vi "sub_peltier 1 control.vi"(0 "Save File":path, 1 "Save Data to File":bool caption="Save?", 3 "COM":i16, 4 "Array #":i32) -> ()   [LabVIEW 2020]
uses:
  <vilib>/Instr/_visa.llb/VISA Find Search Mode.ctl
  <vilib>/Utility/error.llb/DialogType.ctl
  globalvariables.vi
  <vilib>/Utility/file.llb/Write Delimited Spreadsheet (string).vi
  <vilib>/Utility/file.llb/Write Delimited Spreadsheet (DBL).vi
panel:
  in  "Controller Settings":enum32{"Page 1"}(tab)
  in  "Proportional Bandwidth":dbl=50.0
  in  "Integral Gain":dbl
  in  "Derivative Gain":dbl
  in  "Set Limit High":dbl=100.0
  in  "Set Limit Low":dbl=-20.0
  in  "Control Sensor Offset":dbl
  in  "Sample Rate (s)":i16=1
  in  "Alarm Settings":enum32{"Page 1"}(tab)
  in  "Shutdown Output w/ Alarm 2":bool
  in  "Clear Alarm Latch":bool
  in  "Shutdown Output w/ Alarm 1":bool
  in  "Alarm 2 Deadband":dbl
  in  "Alarm 2 Low":dbl
  in  "Alarm 2 High":dbl=60.0
  in  "Alarm 1 Deadband":dbl
  in  "Alarm 1 Low":dbl
  in  "Alarm 1 High":dbl=60.0
  in  "Alarm Latch":T1(radio)
  out "Alarm":bool
  in  "Graph Data":enum32{"Tab 1"}(tab)
  in  "About":bool
  out "Elapsed Time":dbl=-3262346310.140625
  out "Start Sample Time":timestamp=timestamp(3262346310.140625 s since 1904-01-01)
  out "Sample in Time":timestamp
  in  "Strip Chart 2":T2={"TEMPERATURE"=36.2, "Value"=-16.0, "Value 2"=-13.8}
  out "Set Temperature":dbl
  out "Input 2 Sensor":dbl
  out "Control Sensor":dbl
  in  "Misc Settings":enum32{"Page 1"}(tab)
  in  "Analog Output Multiplier":dbl=1.0
  in  "Sensor Type":enum32{"15K", "10K"}(radio)=enum."10K"
  in  "Output Polarity":enum32{"Cool", "Heat "}(radio)
  in  "EEPROM Write Enable":bool
  in  "Temperature 2 Display":T3(radio)=enum."Radio Selection 3"
  out "Firmware Version":string
  out "CRC Error":bool
  out "error out":errorcluster
  out "Reading Configuration":sgl
  in  "Tab Control":enum32{"Page 1"}(tab)
  out "Power":i16(slide) scale=0.0..100.0
  out "Strip Chart":T2(graph)
  out "Sampling":bool
  in  "Run Peltier":bool
  # "%"
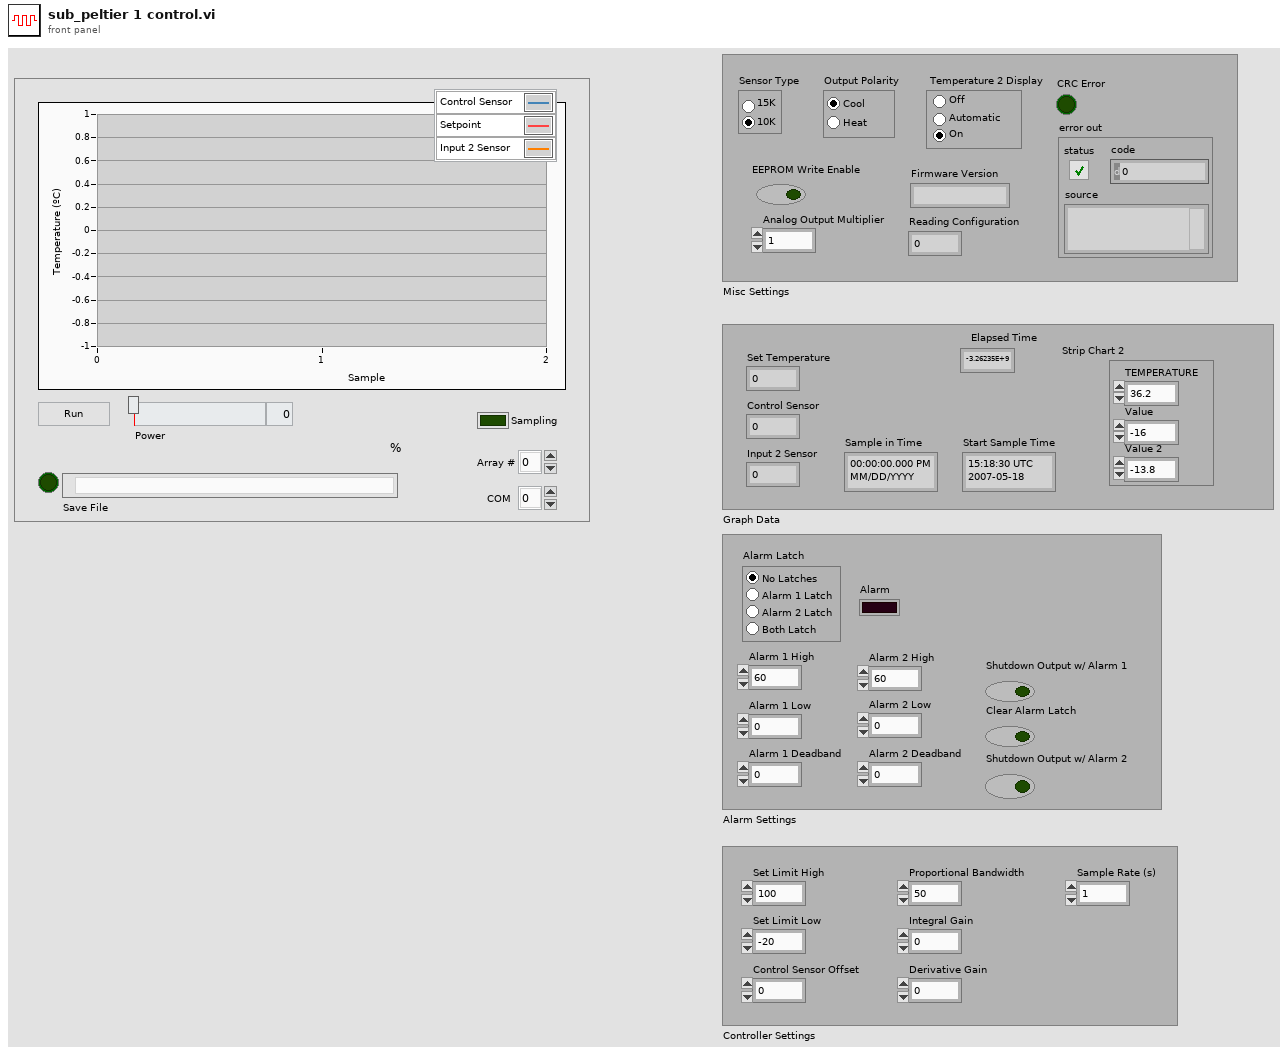
[diagram p1: front panel]
types:
  T1 = enum32{"Radio Selection 1", "Radio Selection 2", "Radio Selection 3", "Radio Selection 4"}
  T2 = cluster{"TEMPERATURE":dbl, "Value":dbl, "Value 2":dbl}
  T3 = enum32{"Radio Selection 1", "Radio Selection 2", "Radio Selection 3"}
  T4 = cluster{"Read Model":bool, "Read Settings":bool, "Read Controls":bool, "Sample":bool, "Start":bool, "End":bool, "CRC Error":bool}
  T5 = typedef "VISA Find Search Mode.ctl" = u32
  T6 = cluster{"TEMPERATURE":dbl, "Value":dbl, "Value 2":dbl}[]
  T7 = typedef "DialogType.ctl" = u16
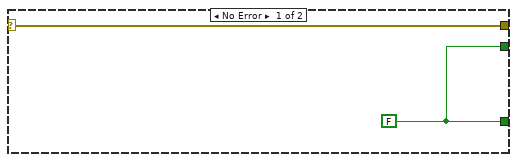
[diagram p2: hidden frame]
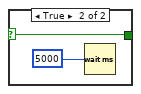
[diagram p3: hidden frame]
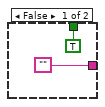
[diagram p4: hidden frame]
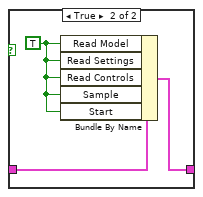
[diagram p10: hidden frame]
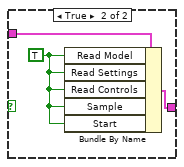
[diagram p12: hidden frame]
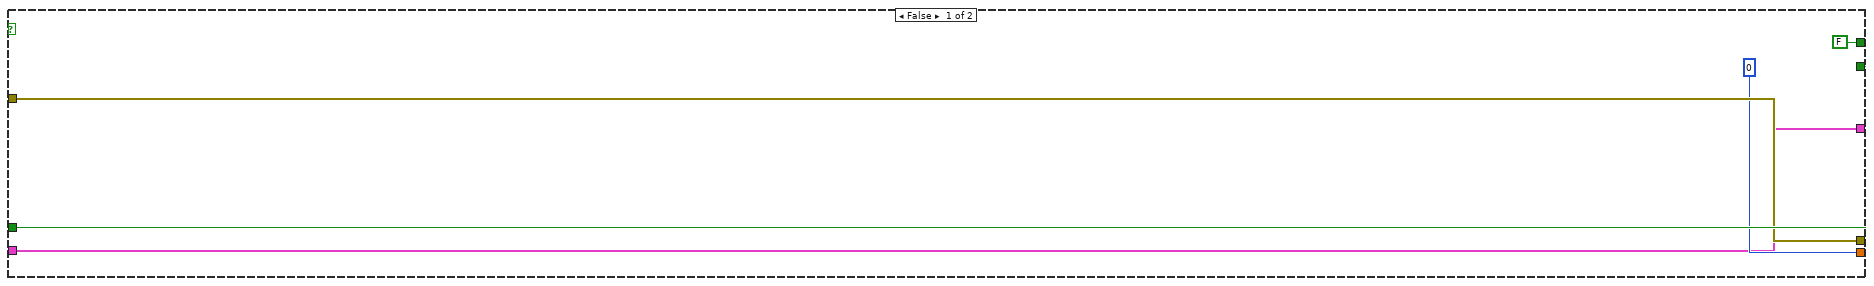
[diagram p13: hidden frame]
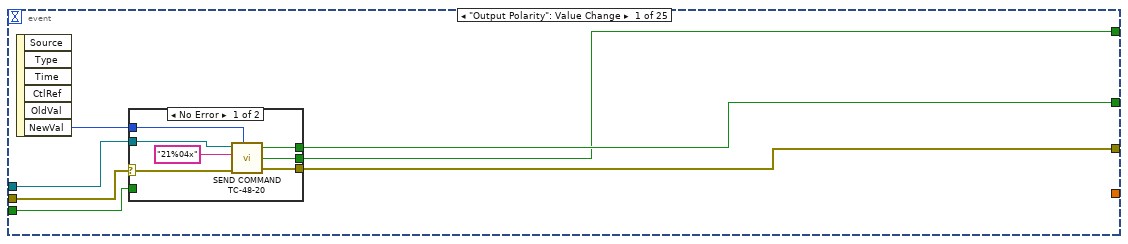
[diagram p16: hidden frame]
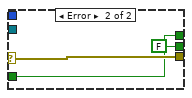
[diagram p17: hidden frame]
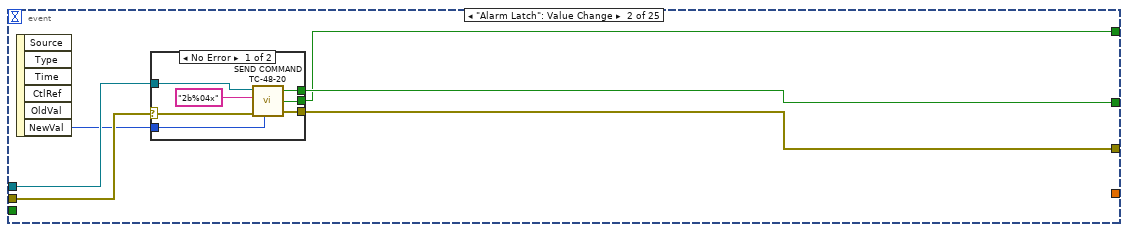
[diagram p18: hidden frame]
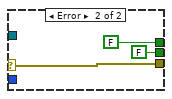
[diagram p19: hidden frame]
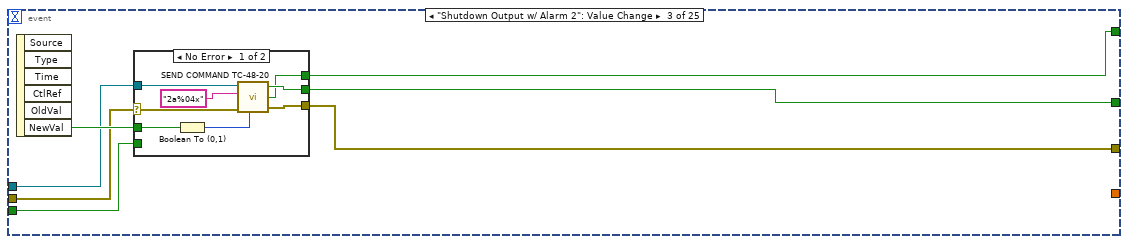
[diagram p20: hidden frame]
diagram:
  w1 = FALSE  # CRC Error
  w2 = FALSE  # End
  w4 = TRUE  # Start
  w5 = TRUE  # Sample
  w6 = TRUE  # Read Controls
  w7 = TRUE  # Read Settings
  w8 = TRUE  # Read Model
  # "CHECK CONTROLS"
  n1 = Bundle("Read Model"=w8, "Read Settings"=w7, "Read Controls"=w6, "Sample"=w5, "Start"=w4, "End"=w2, "CRC Error"=w1) -> (w3:T4)  [unwired: 1 in]
  n2 = while {
    tunnel: [w24] -> w12
    tunnel: [w19] -> w11
    tunnel: errorcluster {"status"=FALSE, "code"=0, "source"=""} ("Startup error in (no error)") -> [w23]
    tunnel: w3 -> [w17]
    tunnel: [w14] -> w10
    stop <- w18 continue-if-true
    # "Connect to Peltier Controller"
    n3 = while {
      tunnel: w23 -> [w46]
      tunnel: [w48] -> w22
      tunnel: [w50] -> w21
      tunnel: [w39] -> w16
      stop <- TRUE stop-if-true
      w55 = u16 0 items=["None", "XON/XOFF", "RTS/CTS", "XON/XOFF & RTS/CTS", "DTR/DSR", "XON/XOFF & DTR/DSR"] ("Serial Settings:Flow Control")
      w51 = u16 0 items=["None", "Odd", "Even", "Mark", "Space"] ("Serial Settings:Parity")
      w56 = T5 4 items=["Canonical Names Only"=0, "Aliases Only"=1, "Include Matching Aliases"=2, "Include All Aliases"=4] ("Search Mode")
      n4 = Greater Than 0?(x="COM") -> (x > 0?=w42:bool)
      n5 = property on="Firmware Version" class="Str"("Value"="") -> ()  [unwired: 2 in, 2 out]
      n6 = case shown="True" w42 {
        tunnel: "COM" -> [_ w63]
        tunnel: ["" w60] -> w40
        tunnel: [TRUE FALSE] -> w39
        frame False {
        }
        frame True {
          n7 = Number To Decimal String(number=w63) -> (decimal integer string=w61:string)  [unwired: 1 in]
          n8 = Concatenate Strings("COM", w61) -> (w60:string)
        }
      }
      n9 = VISA Find Resource(8:w46, 10:w56) -> (0:w49:errorcluster)  [unwired: 1 in, 2 out]
      n10 = Coerce To Type(0:w40, 1:refnum<visa-resource-name> refnum ("SELECT PORT")) -> (2:w43:refnum<visa-resource-name>)
      n11 = property class="Instr" props=["Baud", "Data Bits", "Parity", "Stop Bits", "Flow Cntrl", "Rsrc Name", "Is Connected"](reference=w43, error in=w49, "Baud"=u32 115200 ("Numeric 6"), "Data Bits"=u16 8, "Parity"=w51, "Stop Bits"=u16 10, "Flow Cntrl"=w55) -> (reference out=w50:refnum<visa-resource-name>, error out=w48:errorcluster)  [unwired: 2 out]
    }
    n12 = VISA Set I/O Buffer Size(VISA resource name=w21, error in (no error)=w22) -> (VISA resource name out=w25:refnum<visa-resource-name>, error out=w26:errorcluster)  [unwired: 2 in]
    n13 = VISA Flush I/O Buffer(VISA resource name=w25, error in (no error)=w26) -> (VISA resource name out=w24:refnum<visa-resource-name>, error out=w20:errorcluster)  [unwired: 1 in]
    n14 = case shown="Error" w20 {
      selector: w20 -> [w28 w32]
      tunnel: [w28 w32] -> w19
      tunnel: [w27 w30] -> w18
      tunnel: [w27 w29] -> w15
      frame No Error {
        w27 = FALSE
      }
      frame Error {
        n15 = Two Button Dialog(message=" Unable to communicate with controller (Error 1), check:\n• Controller is ON and correctly wired\n• Correct communications port is selected\n• Another program is not using the communications port ", 1:"EXIT" ("F button name (\"Cancel\")"), 2:"RESTART" ("T button name (\"OK\")")) -> (T button?=w31:bool)
        n16 = case shown="False" w31 {
          selector: w31 -> [w36 w37]
          tunnel: [w36 w37] -> w30
          frame False {
          }
          frame True {
            n17 = Wait (ms)(milliseconds to wait=u32 5000) -> ()  [unwired: 1 out]
          }
        }
        n18 = Not(x=w30) -> (.not. x?=w29:bool)
      }
    }
    n19 = Or(x=w16, y=w15) -> (x .or. y?=w13:bool)
    n20 = Bundle By Name(cluster=w17, "End"=w13) -> (w14:T4)
  }
  n21 = while {
    shift-right: [w64] -> _
    shift-left: w10 -> [w75]
    tunnel: w12 -> [w96]
    tunnel: w11 -> [w83]
    i -> [w65]
    stop <- w77 stop-if-true
    # "VARIABLES"
    # "ERROR PROCESSING"
    # "CONTINUE OR STOP WITH ERROR FROM CRC?"
    n22 = global read "globalvariables.vi" "Peltier Update"() -> (w81:bool[])
    n23 = Bundle By Name(cluster=w75, "CRC Error"=FALSE) -> (w76:T4)
    n24 = property on="Array #" class="DigNum (strict)"() -> ("Value"=w79:i32)  [unwired: 2 in, 2 out]
    n25 = Index Array(array=w81, index=w79) -> (element=w80:bool)
    n26 = case shown="True" w80 {
      tunnel: w76 -> [w105 w108]
      tunnel: [w105 w107] -> w78
      frame False {
      }
      frame True {
        n27 = global read "globalvariables.vi" "Peltier Set Temp"() -> (w115:dbl[])
        n28 = global read "globalvariables.vi" "Peltier Update"() -> (w113:bool[])
        n29 = global read "globalvariables.vi" "Peltier Stop"() -> (w106:bool)
        n30 = property on="Array #" class="DigNum (strict)"() -> ("Value"=w112:i32)  [unwired: 2 in, 2 out]
        n31 = global read "globalvariables.vi" "Peltier Save"() -> (w109:bool)
        n32 = case shown="True" w106 {
          selector: w106 -> [_ w118]
          tunnel: w108 -> [w116 w120]
          tunnel: [w116 w119] -> w107
          frame False {
          }
          frame True {
            n33 = Bundle By Name(cluster=w120, "End"=w118) -> (w119:T4)
            n34 = property on="Run Peltier" class="Bool (strict)"("Value"=FALSE ("Run Peltier")) -> ()  [unwired: 2 in, 2 out]
          }
        }
        n35 = Index Array(array=w115, index=w112) -> (element=w114:dbl)
        n36 = Replace Array Subset(array=w113, new element=FALSE ("Is Peltier Command Ready?"), index=w112) -> (w110:bool[])
        n37 = property on="Save Data to File" class="Bool (strict)"("Value"=w109) -> ()  [unwired: 2 in, 2 out]
        n38 = global write "globalvariables.vi" "Peltier Update"(w110) -> ()
        n39 = property on="Set Temperature" class="DigNum (strict)"("Val(Sgnl)"=w114) -> ()  [unwired: 2 in, 2 out]
      }
    }
    n40 = flat-sequence {
      tunnel: [w1279] -> w95
      tunnel: [w1278] -> w94
      tunnel: [w1277] -> w93
      tunnel: w78 -> [w1276]
      tunnel: w96 -> [w1273]
      tunnel: w83 -> [w1272]
      tunnel: w95 -> [w1389]
      tunnel: w94 -> [w1395]
      tunnel: w93 -> [w1394]
      tunnel: [w1391] -> w87
      tunnel: [w1390] -> w85
      tunnel: [w1388] -> w89
      frame #0 {
        n41 = Unbundle By Name(w1276) -> ("Start"=w1274:bool, "Read Model"=w1271:bool)
        n42 = Or(x=w1274, y=w1271) -> (x .or. y?=w1275:bool)
        n43 = case shown="True" w1275 {
          tunnel: [w1282 w1289] -> w1279
          tunnel: [w1281 w1288] -> w1278
          tunnel: [w1280 w1287] -> w1277
          tunnel: w1272 -> [w1282 w1285]
          tunnel: w1276 -> [w1280 w1286]
          tunnel: w1273 -> [w1281 w1284]
          tunnel: w1271 -> [_ w1283]
          frame False {
          }
          frame True {
            # "START"
            # "READ MODEL"
            n44 = case shown="No Error" w1285 {
              selector: w1285 -> [w1291 w1385]
              tunnel: [w1296 w1385] -> w1289
              tunnel: [w1295 w1384] -> w1288
              tunnel: [w1294 w1383] -> w1287
              tunnel: w1284 -> [w1293 w1384]
              tunnel: w1286 -> [w1292 w1383]
              tunnel: w1283 -> [w1290 _]
              frame No Error {
                n45 = case shown="True" w1290 {
                  tunnel: [w1297 w1301] -> w1296
                  tunnel: [w1298 w1303] -> w1295
                  tunnel: w1292 -> [w1299 w1305]
                  tunnel: [w1299 w1304] -> w1294
                  tunnel: w1293 -> [w1298 w1303]
                  tunnel: w1291 -> [w1297 w1300]
                  frame False {
                  }
                  frame True {
                    n46 = while {
                      tunnel: w1305 -> [w1314]
                      tunnel: [w1326] -> w1304
                      tunnel: w1303 -> [w1316]
                      tunnel: [w1318] -> w1301
                      tunnel: w1300 -> [w1309]
                      i -> [w1322]
                      stop <- w1320 stop-if-true
                      n47 = Greater Or Equal?(x=w1322, y=3) -> (x >= y?=w1321:bool)
                      n48 = case shown="False" w1321 {
                        tunnel: w1314 -> [w1332 w1336]
                        tunnel: [w1332 w1335] -> w1312
                        tunnel: [FALSE ("true") w1333] -> w1306
                        frame False {
                        }
                        frame True {
                          n49 = One Button Dialog(message="Commuincation Error") -> (true=w1333:bool)  [unwired: 1 in]
                          n50 = Bundle By Name(cluster=w1336, "End"=w1333) -> (w1335:T4)
                        }
                      }
                      n51 = call "QUERY MODEL9613.vi"("Communications Port"=w1316) -> ("error out"=w1310:errorcluster, "CRC ERROR"=w1313:bool, "CONTROLLER MODEL"=w1319:string)  [unwired: 3 in]
                      n52 = Wait Until Next ms Multiple(millisecond multiple=120) -> ()  [unwired: 1 out]
                      n53 = Unbundle By Name(w1309) -> ("status"=w1317:bool)
                      n54 = Merge Errors(w1309, w1310) -> (w1318:errorcluster)
                      n55 = Not(x=w1317) -> (.not. x?=w1307:bool)
                      n56 = Equal?(x=w1319, y="9613") -> (x = y?=w1308:bool)
                      n57 = And(x=w1307, y=w1308) -> (x .and. y?=w1315:bool)
                      n58 = Compound Arithmetic op=OR(w1315, w1313, w1306) -> (w1320:bool)
                      n59 = case shown="True" w1313 {
                        selector: w1313 -> [_ w1329]
                        tunnel: w1312 -> [w1327 w1330]
                        tunnel: [w1327 w1328] -> w1311
                        frame False {
                        }
                        frame True {
                          n60 = Bundle By Name(cluster=w1330, "CRC Error"=w1329) -> (w1328:T4)
                        }
                      }
                      n61 = case shown="True" w1315 {
                        tunnel: [w1340 w1350] -> w1326
                        tunnel: w1316 -> [_ w1348]
                        tunnel: w1311 -> [w1337 w1341]
                        frame False {
                          w1338 = FALSE
                          n62 = Bundle By Name(cluster=w1337, "Read Model"=TRUE, "Read Settings"=w1338, "Read Controls"=w1338, "Sample"=w1338, "Start"=w1338) -> (w1340:T4)
                        }
                        frame True {
                          w1349 = FALSE
                          n63 = call "QUERY FIRMWARE VERSION M9613.vi"("Communications Port"=w1348) -> ("error out"=w1347:errorcluster, "VERSION NUMBER"=w1345:u32)  [unwired: 8 in, 1 out]
                          n64 = case shown="No Error" w1347 {
                            tunnel: w1345 -> [w1354 _]
                            tunnel: [w1353 ""] -> w1342
                            frame No Error {
                              n65 = case shown="21" w1354 {
                                tunnel: ["B" "C" "D" "E" "F" "G" "H" "I" "J" "K" "L" "M" "N" "O" "P" "Q" "R" "S" "T" "U" "V" "W" "X" "Y" "Z" "" "A"] -> w1353
                                frame 2 {
                                }
                                frame 3 {
                                }
                                frame 4 {
                                }
                                frame 5 {
                                }
                                frame 6 {
                                }
                                frame 7 {
                                }
                                frame 8 {
                                }
                                frame 9 {
                                }
                                frame 10 {
                                }
                                frame 11 {
                                }
                                frame 12 {
                                }
                                frame 13 {
                                }
                                frame 14 {
                                }
                                frame 15 {
                                }
                                frame 16 {
                                }
                                frame 17 {
                                }
                                frame 18 {
                                }
                                frame 19 {
                                }
                                frame 20 {
                                }
                                frame 21 {
                                }
                                frame 22 {
                                }
                                frame 23 {
                                }
                                frame 24 {
                                }
                                frame 25 {
                                }
                                frame 26 {
                                }
                                frame 0, Default {
                                }
                                frame 1 {
                                }
                              }
                            }
                            frame Error {
                            }
                          }
                          "Firmware Version" <- w1342
                          n66 = Greater Or Equal?(x=w1345, y=u32 8) -> (x >= y?=w1343:bool)
                          n67 = case shown="True" w1343 {
                            tunnel: [u8 2 u8 0] -> w1344
                            frame False {
                            }
                            frame True {
                            }
                          }
                          n68 = property on="EEPROM Write Enable" class="Bool (strict)"("Disabled"=w1344) -> ()  [unwired: 2 in, 2 out]
                          n69 = Bundle By Name(cluster=w1341, "Read Model"=w1349, "Start"=w1349) -> (w1350:T4)
                        }
                      }
                    }
                    n70 = property on="Strip Chart" class="WFChart (strict)"("History Data"=T6 []) -> ()  [unwired: 2 in, 2 out]
                  }
                }
              }
              frame Error {
              }
            }
          }
        }
      }
      frame #1 {
        # "READ SETTINGS"
        n71 = Unbundle By Name(w1394) -> ("Read Settings"=w1386:bool)
        n72 = Unbundle By Name(w1389) -> ("status"=w1393:bool)
        n73 = Not(x=w1393) -> (.not. x?=w1387:bool)
        n74 = And(x=w1387, y=w1386) -> (x .and. y?=w1392:bool)
        n75 = case shown="No Error" w1389 {
          selector: w1389 -> [w1396 w1621]
          tunnel: w1395 -> [w1402 w1622]
          tunnel: w1394 -> [w1401 w1625]
          tunnel: w1392 -> [w1400 _]
          tunnel: [w1399 w1624] -> w1391
          tunnel: [w1398 w1621] -> w1390
          tunnel: [w1397 w1622] -> w1388
          frame No Error {
            n76 = case shown="True" w1400 {
              tunnel: w1396 -> [w1405 w1414]
              tunnel: w1402 -> [w1403 w1411]
              tunnel: w1401 -> [w1406 w1408]
              tunnel: [w1406 w1413] -> w1399
              tunnel: [w1405 w1412] -> w1398
              tunnel: [w1403 w1410] -> w1397
              frame False {
                n77 = property on="Reading Configuration" class="DigNum (strict)"("Value"=0) -> ()  [unwired: 2 in, 2 out]
              }
              frame True {
                n78 = while {
                  tunnel: w1411 -> [w1426]
                  tunnel: w1414 -> [w1434]
                  tunnel: [w1425] -> w1412
                  tunnel: [w1426] -> w1410
                  tunnel: w1408 -> [w1419]
                  tunnel: [w1416] -> w1407
                  i -> [w1420]
                  stop <- w1433 stop-if-true
                  n79 = case shown="0, Default" w1420 {
                    tunnel: w1426 -> [w1450 w1456 w1465 w1472 w1480 w1485 w1496 w1505 w1522 w1528 w1536 w1543 w1552 w1562 w1575 w1580 w1590 w1596 w1604 w1613 w1618]
                    tunnel: w1434 -> [w1446 w1455 w1462 w1470 w1479 w1483 w1495 w1499 w1521 w1525 w1533 w1540 w1547 w1561 w1574 w1582 w1587 w1597 w1603 w1612 w1619]
                    tunnel: [w1449 _ _ _ w1475 _ _ _ _ _ _ _ _ _ _ _ _ _ _ _ _] -> w1423
                    tunnel: [w1445 w1453 w1461 w1468 w1477 w1484 w1493 w1500 w1517 w1526 w1532 w1539 w1546 w1563 w1576 w1583 w1588 w1593 w1600 w1607 w1617] -> w1432
                    selector: w1420 -> [w1445 w1453 w1461 w1468 w1477 w1484 w1493 w1500 w1517 w1526 w1532 w1539 w1546 w1563 w1576 w1583 w1588 w1593 w1600 w1607 w1617]
                    tunnel: [w1445 w1453 w1461 w1468 w1477 w1484 w1493 w1500 w1517 w1526 w1532 w1539 w1546 w1563 w1576 w1583 w1588 w1593 w1600 w1607 w1617] -> w1421
                    tunnel: [FALSE ("CRC") w1451 w1459 w1467 FALSE ("CRC") w1481 w1489 w1498 w1509 w1523 w1531 w1538 w1544 w1555 w1568 w1578 w1585 w1591 w1598 w1605 w1615] -> w1418
                    tunnel: [w1448 w1454 w1464 w1471 w1478 w1486 w1494 w1504 w1514 w1527 w1535 w1542 w1551 w1559 w1572 w1581 w1589 w1594 w1602 w1611 w1620] -> w1427
                    tunnel: [w1444 w1452 w1460 w1466 w1474 w1482 w1488 w1497 w1510 w1524 w1530 w1537 w1545 w1556 w1569 w1577 w1584 w1592 w1599 w1606 w1614] -> w1417
                    frame 0, Default {
                      n80 = call "QUERY INPUT 1 M9613.vi"("Communications Port"=w1450, "error in"=w1446) -> ("CRC ERROR"=w1444:bool, "TEMPERATURE"=w1447:dbl, "error out"=w1448:errorcluster)
                      n81 = property on="Control Sensor" class="DigNum (strict)"("Value"=w1447) -> ()  [unwired: 2 in, 2 out]
                      n82 = property on="Power" class="Slide (strict)"() -> ("Value"=w1449:i16)  [unwired: 2 in, 2 out]
                    }
                    frame 1 {
                      n83 = call "QUERY ALARMS M9613.vi"("Communications Port"=w1456, "error in"=w1455) -> ("CRC ERROR"=w1452:bool, "End"=w1451:bool, "ALARM VALUE"=w1457:dbl, "error out"=w1454:errorcluster)
                      n84 = Not Equal To 0?(x=w1457) -> (x != 0?=→"Alarm":bool)
                    }
                    frame 2 {
                      n85 = call "QUERY CONTROL MODE M9613.vi"("Communications Port"=w1465, "error in"=w1462) -> ("CRC ERROR"=w1460:bool, "End"=w1459:bool, "CONTROL MODE"=w1463:dbl, "error out"=w1464:errorcluster)
                      n86 = property on="Output Polarity" class="RadioBtnsControl (strict)"("Value"=w1463) -> ()  [unwired: 2 in, 2 out]
                    }
                    frame 3 {
                      n87 = call "QUERY ALARM LATCH SETTING M9613.vi"("Communications Port"=w1472, "error in"=w1470) -> ("CRC ERROR"=w1466:bool, "End"=w1467:bool, "ALARM LATCH SETTING"=w1469:dbl, "error out"=w1471:errorcluster)
                      n88 = property on="Alarm Latch" class="RadioBtnsControl (strict)"("Value"=w1469) -> ()  [unwired: 2 in, 2 out]
                    }
                    frame 4 {
                      n89 = call "QUERY POWER OUT M9613.vi"("Communications Port"=w1480, "error in"=w1479) -> ("CRC ERROR"=w1474:bool, "POWER OUT, %"=w1476:dbl, "error out"=w1478:errorcluster)
                      n90 = To Word Integer(number=w1476) -> (16bit integer=w1475:i16)
                    }
                    frame 5 {
                      n91 = call "QUERY SETPOINT M9613.vi"("Communications Port"=w1485, "error in"=w1483) -> ("CRC ERROR"=w1482:bool, "End"=w1481:bool, "SET POINT"=w1487:dbl, "error out"=w1486:errorcluster)
                      n92 = property on="Set Temperature" class="DigNum (strict)"("Value"=w1487) -> ()  [unwired: 2 in, 2 out]
                    }
                    frame 6 {
                      n93 = call "QUERY ALARM 2 STATUS M9613.vi"("Communications Port"=w1496, "error in"=w1495) -> ("CRC ERROR"=w1488:bool, "End"=w1489:bool, "ALARM 2 OUTPUT STATUS"=w1490:dbl, "error out"=w1494:errorcluster)
                      n94 = Number To Boolean Array(number=w1490) -> (Boolean array=w1492:bool[])
                      n95 = Or Array Elements(Boolean array=w1492) -> (logical OR=w1491:bool)
                      n96 = property on="Shutdown Output w/ Alarm 2" class="Bool (strict)"("Value"=w1491) -> ()  [unwired: 2 in, 2 out]
                    }
                    frame 7 {
                      n97 = call "QUERY ALARM 1 STATUS M9613.vi"("Communications Port"=w1505, "error in"=w1499) -> ("CRC ERROR"=w1497:bool, "End"=w1498:bool, "ALARM 2 OUTPUT STATUS"=w1503:dbl, "error out"=w1504:errorcluster)
                      n98 = Number To Boolean Array(number=w1503) -> (Boolean array=w1502:bool[])
                      n99 = Or Array Elements(Boolean array=w1502) -> (logical OR=w1501:bool)
                      n100 = property on="Shutdown Output w/ Alarm 1" class="Bool (strict)"("Value"=w1501) -> ()  [unwired: 2 in, 2 out]
                    }
                    frame 8 {
                      n101 = call "QUERY PROPORTIONAL BW M9613.vi"("Communications Port"=w1522, "error in"=w1521) -> ("CRC ERROR"=w1513:bool, "End"=w1508:bool, "PROPOTIONAL BW"=w1518:dbl, "error out"=w1516:errorcluster)
                      n102 = call "QUERY INTEGRAL GAIN M9613.vi"("Communications Port"=w1522, "error in"=w1516) -> ("CRC ERROR"=w1512:bool, "End"=w1507:bool, "INTEGRAL GAIN"=w1519:dbl, "error out"=w1515:errorcluster)
                      n103 = call "QUERY DERIVATIVE GAIN M9613.vi"("Communications Port"=w1522, "error in"=w1515) -> ("CRC ERROR"=w1511:bool, "End"=w1506:bool, "DERIVATIVE GAIN"=w1520:dbl, "error out"=w1514:errorcluster)
                      n104 = property on="Proportional Bandwidth" class="DigNum (strict)"("Value"=w1518) -> ()  [unwired: 2 in, 2 out]
                      n105 = property on="Integral Gain" class="DigNum (strict)"("Value"=w1519) -> ()  [unwired: 2 in, 2 out]
                      n106 = property on="Derivative Gain" class="DigNum (strict)"("Value"=w1520) -> ()  [unwired: 2 in, 2 out]
                      n107 = Compound Arithmetic op=OR(w1513, w1512, w1511) -> (w1510:bool)
                      n108 = Compound Arithmetic op=OR(w1508, w1507, w1506) -> (w1509:bool)
                    }
                    frame 9 {
                      n109 = call "INPUT 1 SENSOR OFFSET M9613.vi"("Communications Port"=w1528, "error in"=w1525) -> ("CRC ERROR"=w1524:bool, "End"=w1523:bool, "INPUT 1 SENSOR OFFSET"=w1529:dbl, "error out"=w1527:errorcluster)
                      n110 = property on="Control Sensor Offset" class="DigNum (strict)"("Value"=w1529) -> ()  [unwired: 2 in, 2 out]
                    }
                    frame 10 {
                      n111 = call "QUERY ALARM LATCH SETTING M9613.vi"("Communications Port"=w1536, "error in"=w1533) -> ("CRC ERROR"=w1530:bool, "End"=w1531:bool, "ALARM LATCH SETTING"=w1534:dbl, "error out"=w1535:errorcluster)
                      n112 = property on="Alarm Latch" class="RadioBtnsControl (strict)"("Value"=w1534) -> ()  [unwired: 2 in, 2 out]
                    }
                    frame 11 {
                      n113 = call "QUERY SENSOR TYPE M9613.vi"("Communications Port"=w1543, "error in"=w1540) -> ("CRC ERROR"=w1537:bool, "End"=w1538:bool, "SENSOR TYPE"=w1541:dbl, "error out"=w1542:errorcluster)
                      n114 = property on="Sensor Type" class="RadioBtnsControl (strict)"("Value"=w1541) -> ()  [unwired: 2 in, 2 out]
                    }
                    frame 12 {
                      n115 = call "QUERY ALARM 1 DEADBAND M9613.vi"("Communications Port"=w1552, "error in"=w1547) -> ("CRC ERROR"=w1545:bool, "End"=w1544:bool, "ALARM 1 DEADBAND"=w1549:dbl, "error out"=w1551:errorcluster)
                      n116 = Divide(x=w1549, y=10.0) -> (x/y=w1550:dbl)
                      n117 = property on="Alarm 1 Deadband" class="DigNum (strict)"("Value"=w1550) -> ()  [unwired: 2 in, 2 out]
                    }
                    frame 13 {
                      n118 = call "QUERY HIGH ALARM SET POINT M9613.vi"("Communications Port"=w1562, "error in"=w1561) -> ("CRC ERROR"=w1554:bool, "HIGH ALARM SETPOINT INPUT 1"=w1557:dbl, "error out"=w1560:errorcluster)
                      n119 = call "QUERY LOW ALARM SET POINT M9613.vi"("Communications Port"=w1562, "error in"=w1560) -> ("CRC ERROR"=w1553:bool, "End"=w1555:bool, "LOW ALARM SETPOINT"=w1558:dbl, "error out"=w1559:errorcluster)
                      n120 = Or(x=w1554, y=w1553) -> (x .or. y?=w1556:bool)
                      n121 = property on="Alarm 1 High" class="DigNum (strict)"("Value"=w1557) -> ()  [unwired: 2 in, 2 out]
                      n122 = property on="Alarm 1 Low" class="DigNum (strict)"("Value"=w1558) -> ()  [unwired: 2 in, 2 out]
                    }
                    frame 14 {
                      n123 = call "QUERY HIGH ALARM SET POINT INPUT 2 M9613.vi"("Communications Port"=w1575, "error in"=w1574) -> ("CRC ERROR"=w1567:bool, "End"=w1566:bool, "HIGH ALARM SETPOINT INPUT 2"=w1571:dbl, "error out"=w1573:errorcluster)
                      n124 = call "QUERY LOW ALARM SET POINT INPUT 2 M9613.vi"("Communications Port"=w1575, "error in"=w1573) -> ("CRC ERROR"=w1565:bool, "End"=w1564:bool, "LOW ALARM SETPOINT INPUT 2"=w1570:dbl, "error out"=w1572:errorcluster)
                      n125 = Or(x=w1567, y=w1565) -> (x .or. y?=w1569:bool)
                      n126 = Or(x=w1566, y=w1564) -> (x .or. y?=w1568:bool)
                      n127 = property on="Alarm 2 High" class="DigNum (strict)"("Value"=w1571) -> ()  [unwired: 2 in, 2 out]
                      n128 = property on="Alarm 2 Low" class="DigNum (strict)"("Value"=w1570) -> ()  [unwired: 2 in, 2 out]
                    }
                    frame 15 {
                      n129 = call "QUERY ANALOG OUTPUT MULTIPLIER M9613.vi"("Communications Port"=w1580, "error in"=w1582) -> ("CRC ERROR"=w1577:bool, "End"=w1578:bool, "ANALOG OUTPUT MULTIPLIER"=w1579:dbl, "error out"=w1581:errorcluster)
                      n130 = property on="Analog Output Multiplier" class="DigNum (strict)"("Value"=w1579) -> ()  [unwired: 2 in, 2 out]
                    }
                    frame 16 {
                      n131 = call "QUERY TEMP 2 DISPLAY M9613.vi"("Communications Port"=w1590, "error in"=w1587) -> ("CRC ERROR"=w1584:bool, "End"=w1585:bool, "TEMPERATURE 2 DISPLAY"=w1586:dbl, "error out"=w1589:errorcluster)
                      n132 = property on="Temperature 2 Display" class="RadioBtnsControl (strict)"("Value"=w1586) -> ()  [unwired: 2 in, 2 out]
                    }
                    frame 17 {
                      n133 = call "QUERY LOW SET RANGE M9613.vi"("Communications Port"=w1596, "error in"=w1597) -> ("CRC ERROR"=w1592:bool, "End"=w1591:bool, "LOW SET RANGE"=w1595:dbl, "error out"=w1594:errorcluster)
                      n134 = property on="Set Limit Low" class="DigNum (strict)"("Value"=w1595) -> ()  [unwired: 2 in, 2 out]
                    }
                    frame 18 {
                      n135 = call "QUERY HIGH SET RANGE M9613.vi"("Communications Port"=w1604, "error in"=w1603) -> ("CRC ERROR"=w1599:bool, "End"=w1598:bool, "HIGH SET RANGE"=w1601:dbl, "error out"=w1602:errorcluster)
                      n136 = property on="Set Limit High" class="DigNum (strict)"("Value"=w1601) -> ()  [unwired: 2 in, 2 out]
                    }
                    frame 19 {
                      n137 = call "QUERY OUTPUT ON M9613.vi"("Communications Port"=w1613, "error in"=w1612) -> ("CRC ERROR"=w1606:bool, "End"=w1605:bool, "OUTPUT ENABLE"=w1610:i8, "error out"=w1611:errorcluster)
                      n138 = Number To Boolean Array(number=w1610) -> (Boolean array=w1609:bool[])
                      n139 = Or Array Elements(Boolean array=w1609) -> (logical OR=w1608:bool)
                      n140 = property on="Run Peltier" class="Bool (strict)"("Value"=w1608) -> ()  [unwired: 2 in, 2 out]
                    }
                    frame 20 {
                      n141 = call "QUERY EEPROM WRITE ENABLE.vi"("Communications Port"=w1618, "error IO"=w1619) -> ("EEPROM WRITE\nENABLED"=w1616:bool, "End"=w1615:bool, "CRC"=w1614:bool, "error IO 2"=w1620:errorcluster)
                      n142 = property on="EEPROM Write Enable" class="Bool (strict)"("Value"=w1616) -> ()  [unwired: 2 in, 2 out]
                    }
                  }
                  "Power" <- w1423
                  n143 = case shown="True" w1418 {
                    selector: w1418 -> [_ w1437]
                    tunnel: w1419 -> [w1435 w1438]
                    tunnel: [w1435 w1436] -> w1415
                    frame False {
                    }
                    frame True {
                      n144 = Bundle By Name(cluster=w1438, "End"=w1437) -> (w1436:T4)
                    }
                  }
                  n145 = case shown="True" w1417 {
                    selector: w1417 -> [_ w1442]
                    tunnel: w1415 -> [w1439 w1440]
                    tunnel: [w1439 w1441] -> w1416
                    tunnel: [w1439 w1440] -> _
                    frame False {
                    }
                    frame True {
                      n146 = Bundle By Name(cluster=w1440, "CRC Error"=w1442) -> (w1441:T4)
                    }
                  }
                  n147 = Divide(x=w1432, y=20) -> (x/y=w1431:dbl)
                  n148 = Equal?(x=w1421, y=20) -> (x = y?=w1433:bool)
                  n149 = Multiply(x=100, y=w1431) -> (x*y=→"Reading Configuration":dbl)
                  n150 = call <vilib>:"Simple Error Handler.vi"("error source (\" \")"="ERROR IN READ CONFIGURATION" ("error source (\" \")"), "error in (no error)"=w1427) -> ("error out"=w1425:errorcluster)  [unwired: 3 in, 4 out]
                }
                n151 = Bundle By Name(cluster=w1407, "Read Settings"=FALSE) -> (w1413:T4)
              }
            }
          }
          frame Error {
            w1623 = TRUE
            n152 = Bundle By Name(cluster=w1625, "Read Model"=w1623, "Read Settings"=w1623) -> (w1624:T4)
          }
        }
      }
    }
    n153 = case shown="Error" w85 {
      selector: w85 -> [w121 w123]
      tunnel: w87 -> [w122 w126]
      tunnel: [w122 w125] -> w86
      tunnel: [w121 w123] -> w84
      frame No Error {
      }
      frame Error {
        n154 = Two Button Dialog(message=" Unable to communicate with controller (Error 2), check:\n• Controller is ON and correctly wired\n• Correct communications port is selected\n• Another program is not using the communications port ", 1:"EXIT" ("F button name (\"Cancel\")"), 2:"RESTART" ("T button name (\"OK\")")) -> (T button?=w124:bool)
        n155 = case shown="False" w124 {
          selector: w124 -> [w133 _]
          tunnel: w126 -> [w132 w134]
          tunnel: [w130 w136] -> w125
          frame False {
            n156 = Not(x=w133) -> (.not. x?=w131:bool)
            n157 = Bundle By Name(cluster=w132, "End"=w131) -> (w130:T4)
          }
          frame True {
            w135 = TRUE
            n158 = Bundle By Name(cluster=w134, "Read Model"=w135, "Read Settings"=w135, "Read Controls"=w135, "Sample"=w135, "Start"=w135) -> (w136:T4)
          }
        }
      }
    }
    n159 = feedback #1() -> (w73:dbl)  [unwired: 1 in]
    n160 = case shown="No Error" w84 {
      selector: w84 -> [w968 w1250]
      tunnel: [w973 w1250] -> w90
      tunnel: w89 -> [w972 _]
      tunnel: w73 -> [w971 _]
      tunnel: w86 -> [w970 w1251]
      tunnel: [w969 w1251] -> w91
      tunnel: w65 -> [w963 _]
      frame No Error {
        # "DISPLAY TEMPERATURE"
        n161 = flat-sequence {
          tunnel: w971 -> [w1000]
          tunnel: w968 -> [w1002]
          tunnel: w972 -> [w999]
          tunnel: [w1001] -> w991
          tunnel: [w997] -> w990
          tunnel: [w998] -> w992
          tunnel: w970 -> [w996]
          tunnel: [w994] -> w989
          tunnel: [w1048] -> w988
          tunnel: [w1047] -> w987
          tunnel: w992 -> [w1045]
          tunnel: w991 -> [w1040]
          tunnel: w990 -> [w1046]
          tunnel: [w1044] -> w986
          tunnel: w989 -> [w1039]
          tunnel: [w1037] -> w985
          tunnel: [w1034] -> w964
          tunnel: w988 -> [w1126]
          tunnel: w987 -> [w1125]
          tunnel: [w1124] -> w984
          tunnel: [w1123] -> w983
          tunnel: w986 -> [w1122]
          tunnel: [w1117] -> w982
          tunnel: w985 -> [w1121]
          tunnel: [w1121] -> w981
          tunnel: [w1120] -> w965
          tunnel: w964 -> [w1119]
          tunnel: [w1160] -> w980
          tunnel: [w1159] -> w979
          tunnel: w984 -> [w1158]
          tunnel: w983 -> [w1157]
          tunnel: w982 -> [w1156]
          tunnel: [w1156] -> w978
          tunnel: w981 -> [w1154]
          tunnel: [w1153] -> w977
          tunnel: [w1155] -> w966
          tunnel: w965 -> [w1155]
          tunnel: w980 -> [w1182]
          tunnel: w979 -> [w1177]
          tunnel: [w1181] -> w976
          tunnel: [w1175] -> w975
          tunnel: w978 -> [w1176]
          tunnel: w977 -> [w1179]
          tunnel: [w1179] -> w974
          tunnel: [w1178] -> w967
          tunnel: w966 -> [w1178]
          tunnel: [w1196] -> w973
          tunnel: w976 -> [w1201]
          tunnel: w975 -> [w1200]
          tunnel: w974 -> [w1193]
          tunnel: [w1197] -> w969
          tunnel: w967 -> [w1187]
          tunnel: w963 -> [w1190]
          frame #0 {
            # "CHECK ALARM STATUS"
            n162 = case shown="No Error" w1002 {
              selector: w1002 -> [w1020 w1033]
              tunnel: [w1010 w1033] -> w1001
              tunnel: w1000 -> [w1019 w1031]
              tunnel: w999 -> [w1011 w1032]
              tunnel: [w1011 w1032] -> w998
              tunnel: [w1019 w1031] -> w997
              tunnel: [w1016 FALSE] -> w993
              tunnel: w996 -> [w1005 w1029]
              tunnel: [w1006 w1029] -> w995
              frame No Error {
                n163 = call "QUERY ALARMS M9613.vi"("Communications Port"=w1011, "error in"=w1020) -> ("CRC ERROR"=w1008:bool, "End"=w1003:bool, "ALARM VALUE"=w1013:dbl, "error out"=w1018:errorcluster)
                n164 = In Range and Coerce(upper limit=32, x=w1013, lower limit=1) -> (In Range?=w1012:bool)  [unwired: 1 out]
                n165 = call "DECODE ALARM STATUS TC4820.vi"("error in (no error)"=w1018, "ALARM STATUS IN"=w1013) -> ("error out"=w1017:errorcluster, "READ CONTROLLER"=w1016:bool)  [unwired: 1 in, 1 out]
                n166 = property on="Alarm" class="Bool (strict)"("Value"=w1012, "Blinking"=w1012) -> ()  [unwired: 2 in, 2 out]
                n167 = call "QUERY ALARM SETPOINT DIABLE M9613.vi"("Communications Port"=w1011, "error in"=w1017) -> ("CRC Error"=w1009:bool, "error out"=w1010:errorcluster)  [unwired: 1 out]
                n168 = Or(x=w1009, y=w1008) -> (x .or. y?=w1007:bool)
                n169 = case shown="True" w1003 {
                  selector: w1003 -> [_ w1023]
                  tunnel: w1005 -> [w1021 w1024]
                  tunnel: [w1021 w1022] -> w1004
                  frame False {
                  }
                  frame True {
                    n170 = Bundle By Name(cluster=w1024, "End"=w1023) -> (w1022:T4)
                  }
                }
                n171 = case shown="True" w1007 {
                  selector: w1007 -> [_ w1027]
                  tunnel: w1004 -> [w1025 w1028]
                  tunnel: [w1025 w1026] -> w1006
                  frame False {
                  }
                  frame True {
                    n172 = Bundle By Name(cluster=w1028, "CRC Error"=w1027) -> (w1026:T4)
                  }
                }
              }
              frame Error {
              }
            }
            n173 = Bundle By Name(cluster=w995, "Read Settings"=w993) -> (w994:T4)
          }
          frame #1 {
            # "READ TEMPERATURE"
            n174 = case shown="No Error" w1040 {
              selector: w1040 -> [w1058 w1098]
              tunnel: w1046 -> [_ _]
              tunnel: w1045 -> [w1056 w1096]
              tunnel: [w1063 w1098] -> w1042
              tunnel: ["Temperature 2 Display" T3."Radio Selection 1" ("Temperature 2 Display")] -> w1044
              tunnel: [w1061 0.0] -> w1035
              tunnel: [w1056 w1096] -> w1043
              tunnel: w1039 -> [w1053 w1094]
              tunnel: [w1054 w1094] -> w1038
              frame No Error {
                n175 = call "QUERY SETPOINT M9613.vi"("Communications Port"=w1056, "error in"=w1058) -> ("CRC ERROR"=w1060:bool, "End"=w1049:bool, "SET POINT"=w1059:dbl, "error out"=w1064:errorcluster)
                n176 = property on="Set Temperature" class="DigNum (strict)"("Value"=w1059) -> ()  [unwired: 2 in, 2 out]
                n177 = case shown="\"Radio Selection 2\"" "Temperature 2 Display" {
                  tunnel: w1056 -> [_ w1080 w1092]
                  tunnel: w1064 -> [w1077 w1085 w1091]
                  tunnel: [w1077 w1084 w1090] -> w1063
                  tunnel: [w1075 w1079 w1087] -> w1061
                  tunnel: [FALSE w1082 w1089] -> w1057
                  tunnel: [FALSE ("End") w1078 w1086] -> w1050
                  frame "Radio Selection 1", Default {
                    w1075 = 0.0 ("TEMP. SENSOR 2")
                    n178 = property on="Input 2 Sensor" class="DigNum (strict)"("Disabled"=2, "Value"=w1075) -> ()  [unwired: 2 in, 2 out]
                  }
                  frame "Radio Selection 2" {
                    n179 = call "QUERY INPUT 2 M9613.vi"("Communications Port"=w1080, "error in"=w1085) -> ("CRC ERROR"=w1082:bool, "End"=w1078:bool, "SECONDARY SENSOR VALUE"=w1079:dbl, "error out"=w1084:errorcluster)
                    "Input 2 Sensor" <- w1079
                    n180 = Wait Until Next ms Multiple(millisecond multiple=50) -> ()  [unwired: 1 out]
                    n181 = property on="Input 2 Sensor" class="DigNum (strict)"("Disabled"=u8 0) -> ()  [unwired: 2 in, 2 out]
                  }
                  frame "Radio Selection 3" {
                    n182 = call "QUERY INPUT 2 M9613.vi"("Communications Port"=w1092, "error in"=w1091) -> ("CRC ERROR"=w1089:bool, "End"=w1086:bool, "SECONDARY SENSOR VALUE"=w1087:dbl, "error out"=w1090:errorcluster)
                    n183 = Wait Until Next ms Multiple(millisecond multiple=u32 50) -> ()  [unwired: 1 out]
                    n184 = property on="Input 2 Sensor" class="DigNum (strict)"("Value"=w1087, "Disabled"=0) -> ()  [unwired: 2 in, 2 out]
                  }
                }
                n185 = Or(x=w1057, y=w1060) -> (x .or. y?=w1055:bool)
                n186 = Or(x=w1050, y=w1049) -> (x .or. y?=w1051:bool)
                n187 = case shown="True" w1051 {
                  selector: w1051 -> [_ w1067]
                  tunnel: w1053 -> [w1065 w1068]
                  tunnel: [w1065 w1066] -> w1052
                  frame False {
                  }
                  frame True {
                    n188 = Bundle By Name(cluster=w1068, "End"=w1067) -> (w1066:T4)
                  }
                }
                n189 = case shown="True" w1055 {
                  selector: w1055 -> [_ w1071]
                  tunnel: w1052 -> [w1069 w1072]
                  tunnel: [w1069 w1070] -> w1054
                  frame False {
                  }
                  frame True {
                    n190 = Bundle By Name(cluster=w1072, "CRC Error"=w1071) -> (w1070:T4)
                  }
                }
              }
              frame Error {
              }
            }
            n191 = case shown="No Error" w1042 {
              selector: w1042 -> [w1106 w1116]
              tunnel: w1043 -> [w1108 w1114]
              tunnel: [w1107 w1116] -> w1048
              tunnel: [w1105 -inf] -> w1036
              tunnel: [w1108 w1114] -> w1047
              tunnel: w1038 -> [w1101 w1113]
              tunnel: [w1099 w1113] -> w1037
              frame No Error {
                n192 = global read "globalvariables.vi" "Peltier Control Sensor"() -> (w1104:dbl[])
                n193 = call "QUERY INPUT 1 M9613.vi"("Communications Port"=w1108, "error in"=w1106) -> ("CRC ERROR"=w1100:bool, "TEMPERATURE"=w1105:dbl, "error out"=w1107:errorcluster)
                "Control Sensor" <- w1105
                n194 = property on="Array #" class="DigNum (strict)"() -> ("Value"=w1102:i32)  [unwired: 2 in, 2 out]
                n195 = Replace Array Subset(array=w1104, new element=w1105, index=w1102) -> (w1103:dbl[])
                n196 = global write "globalvariables.vi" "Peltier Control Sensor"(w1103) -> ()
                n197 = case shown="True" w1100 {
                  selector: w1100 -> [_ w1111]
                  tunnel: w1101 -> [w1109 w1112]
                  tunnel: [w1109 w1110] -> w1099
                  frame False {
                  }
                  frame True {
                    n198 = Bundle By Name(cluster=w1112, "CRC Error"=w1111) -> (w1110:T4)
                  }
                }
              }
              frame Error {
              }
            }
            n199 = property on="Sampling" class="Bool (strict)"("Value"=TRUE) -> ()  [unwired: 2 in, 2 out]
            n200 = Build Array(w1036, w1035) -> (w1034:dbl[])
          }
          frame #2 {
            n201 = case shown="No Error" w1126 {
              selector: w1126 -> [w1133 w1152]
              tunnel: [w1133 w1152] -> w1124
              tunnel: w1125 -> [w1134 w1151]
              tunnel: [w1134 w1151] -> w1123
              tunnel: w1122 -> [w1132 _]
              tunnel: w1119 -> [w1131 _]
              tunnel: [w1129 -inf] -> w1118
              frame No Error {
                n202 = property on="Set Temperature" class="DigNum (strict)"() -> ("Value"=w1129:dbl)  [unwired: 2 in, 2 out]
                n203 = case shown="\"Radio Selection 2\", \"Radio Selection 3\"" w1132 {
                  tunnel: w1129 -> [w1138 w1148]
                  tunnel: [w1139 w1146] -> w1127
                  tunnel: w1131 -> [w1135 w1143]
                  tunnel: [2 3] -> w1130
                  frame "Radio Selection 1", Default {
                    n204 = Index Array(array=w1135) -> (element=w1136:dbl)  [unwired: 1 in]
                    n205 = Bundle(cluster=T2 {"TEMPERATURE"=0.0, "Value"=0.0, "Value 2"=0.0}, "TEMPERATURE"=w1136, "Value"=w1138) -> (w1139:T2)  [unwired: 1 in]
                  }
                  frame "Radio Selection 2", "Radio Selection 3" {
                    n206 = property on="Strip Chart" class="WFChart (strict)"("YScale.Maximum"=8.0, "YScale.Minimum"=30.0) -> ()  [unwired: 2 in, 2 out]
                    n207 = Index Array(array=w1143) -> (element #1=w1142:dbl, element #2=w1141:dbl)  [unwired: 2 in]
                    n208 = Bundle(cluster="Strip Chart 2", "TEMPERATURE"=w1142, "Value"=w1148, "Value 2"=w1141) -> (w1146:T2)
                  }
                }
                "Strip Chart" <- w1127
                n209 = property on="Strip Chart" class="WFChart (strict)"("LegPlots"=w1130, "YScale.UnitLabel.Text"="CELSIUS" ("Y Scale.Unit Label.Text")) -> ()  [unwired: 2 in, 2 out]
              }
              frame Error {
              }
            }
            n210 = Get Date/Time In Seconds() -> (seconds since 1Jan1904=w1120:timestamp)
            n211 = Build Array (concatenate)(w1119, w1118) -> (w1117:dbl[])
          }
          frame #3 {
            # "READ POWER OUT"
            n212 = case shown="No Error" w1158 {
              selector: w1158 -> [w1167 w1174]
              tunnel: [w1166 w1174] -> w1160
              tunnel: [w1164 0.0] -> w1159
              tunnel: w1157 -> [w1165 _]
              tunnel: w1154 -> [w1163 w1172]
              tunnel: [w1161 w1172] -> w1153
              frame No Error {
                n213 = call "QUERY POWER OUT M9613.vi"("Communications Port"=w1165, "error in"=w1167) -> ("CRC ERROR"=w1162:bool, "POWER OUT, %"=w1164:dbl, "error out"=w1166:errorcluster)
                n214 = case shown="True" w1162 {
                  selector: w1162 -> [_ w1170]
                  tunnel: w1163 -> [w1168 w1171]
                  tunnel: [w1168 w1169] -> w1161
                  frame False {
                  }
                  frame True {
                    n215 = Bundle By Name(cluster=w1171, "CRC Error"=w1170) -> (w1169:T4)
                  }
                }
              }
              frame Error {
              }
            }
          }
          frame #4 {
            # "DISPLAY OUTPUT POWER"
            n216 = case shown="No Error" w1182 {
              selector: w1182 -> [w1185 w1186]
              tunnel: [w1185 w1186] -> w1181
              tunnel: w1177 -> [w1183 _]
              frame No Error {
                n217 = Absolute Value(x=w1183) -> (abs(x)=w1184:dbl)
                n218 = property on="Power" class="Slide (strict)"("Value"=w1184) -> ()  [unwired: 2 in, 2 out]
              }
              frame Error {
              }
            }
            n219 = Build Array (concatenate)(w1176, w1177) -> (w1175:dbl[])
            "Sampling" <- FALSE
          }
          frame #5 {
            n220 = Unbundle By Name(w1193) -> ("CRC Error"=w1192:bool)
            n221 = Not Equal To 0?(x=w1190) -> (x != 0?=w1191:bool)
            n222 = And(x="Save Data to File", y=w1191) -> (x .and. y?=w1188:bool)
            n223 = case shown="True" w1192 {
              selector: w1192 -> [_ w1219]
              tunnel: w1193 -> [w1218 w1221]
              tunnel: [w1218 w1220] -> w1198
              frame False {
              }
              frame True {
                n224 = Bundle By Name(cluster=w1221, "Read Model"=w1219, "Read Settings"=w1219) -> (w1220:T4)
              }
            }
            n225 = case shown="False" w1188 {
              tunnel: w1187 -> [w1202 w1203]
              tunnel: [w1202 w1203] -> _
              frame False {
                "Start Sample Time" <- w1202
              }
              frame True {
              }
            }
            n226 = property on="Start Sample Time" class="AbsTime (strict)"() -> ("Value"=w1199:timestamp)  [unwired: 2 in, 2 out]
            n227 = Subtract(x=w1187, y=w1199) -> (x-y=w1194:dbl)
            "Elapsed Time" <- w1194
            n228 = case shown="True" "Save Data to File" {
              tunnel: w1201 -> [w1222 w1231]
              tunnel: [w1222 w1234] -> w1196
              tunnel: "Save File" -> [_ w1229]
              tunnel: w1200 -> [_ w1235]
              tunnel: w1194 -> [_ w1233]
              frame False {
              }
              frame True {
                n229 = Get File Size(file=w1229, error in=w1231) -> (size (in bytes)=w1232:i64, 0:w1230:errorcluster)  [unwired: 1 out]
                n230 = Build Array (concatenate)(w1233, w1235) -> (w1223:dbl[])
                n231 = Not Equal To 0?(x=w1232) -> (x != 0?=w1228:bool)
                n232 = case shown="No Error" w1230 {
                  selector: w1230 -> [w1237 w1249]
                  tunnel: w1228 -> [w1240 _]
                  tunnel: w1229 -> [w1239 w1248]
                  tunnel: [w1238 w1248] -> w1227
                  tunnel: [w1236 w1249] -> w1224
                  frame No Error {
                    n233 = case shown="False" w1240 {
                      tunnel: w1239 -> [w1243 w1247]
                      tunnel: [w1243 w1247] -> w1238
                      tunnel: w1237 -> [w1244 w1246]
                      tunnel: [w1245 w1246] -> w1236
                      frame False {
                        n234 = call-poly <vilib>:"Write Delimited Spreadsheet.vi"("file path (dialog if empty)"=w1243, "2D data"=string[][] [["Time", "T_1", "T_2", "T_Set", "Power"], ["[s]", "[C]", "[C]", "[C]", "[%]"]], "error in (no error)"=w1244, "delimiter (\\t)"="," ("delimiter (\\t)")) -> ("error out"=w1245:errorcluster)  [unwired: 10 in, 1 out]
                      }
                      frame True {
                      }
                    }
                  }
                  frame Error {
                  }
                }
                n235 = call-poly <vilib>:"Write Delimited Spreadsheet.vi"("file path (dialog if empty)"=w1227, "1D data"=w1223, "append to file? (new file:F)"=TRUE, "error in (no error)"=w1224, "delimiter (\\t)"="," ("delimiter (\\t)")) -> ("error out"=w1234:errorcluster)  [unwired: 9 in, 1 out]
              }
            }
            n236 = case shown="Error" w1196 {
              tunnel: w1198 -> [w1204 w1207]
              tunnel: [w1204 w1206] -> w1197
              frame No Error {
              }
              frame Error {
                n237 = Two Button Dialog(message=" Unable to communicate with controller (Error 4), check:\n• Controller is ON and correctly wired\n• Correct communications port is selected\n• Another program is not using the communications port ", 1:"EXIT" ("F button name (\"Cancel\")"), 2:"RESTART" ("T button name (\"OK\")")) -> (T button?=w1205:bool)
                n238 = case shown="False" w1205 {
                  selector: w1205 -> [w1213 _]
                  tunnel: w1207 -> [w1211 w1215]
                  tunnel: [w1212 w1217] -> w1206
                  frame False {
                    n239 = Not(x=w1213) -> (.not. x?=w1214:bool)
                    n240 = Bundle By Name(cluster=w1211, "End"=w1214) -> (w1212:T4)
                  }
                  frame True {
                    w1216 = TRUE
                    n241 = Bundle By Name(cluster=w1215, "Read Model"=w1216, "Read Settings"=w1216, "Read Controls"=w1216, "Sample"=w1216, "Start"=w1216) -> (w1217:T4)
                  }
                }
              }
            }
            "Sample in Time" <- w1187
          }
        }
      }
      frame Error {
      }
    }
    n242 = case shown="No Error" w90 {
      selector: w90 -> [w156 w961]
      tunnel: w89 -> [w162 _]
      tunnel: [w161 0] -> w92
      tunnel: [w160 w961] -> w88
      tunnel: [w155 FALSE] -> w72
      tunnel: w91 -> [w158 w962]
      tunnel: [w157 w962] -> w71
      tunnel: [w153 FALSE ("End")] -> w66
      frame No Error {
        n243 = case shown="True" TRUE {
          tunnel: [w167 w169] -> w155
          tunnel: [w166 w176] -> w160
          tunnel: FALSE -> [w167 w175]
          tunnel: w156 -> [w166 w174]
          tunnel: w162 -> [_ w173]
          tunnel: [0 w172] -> w161
          tunnel: w158 -> [w164 w171]
          tunnel: [w164 w170] -> w157
          tunnel: [FALSE ("End") w168] -> w153
          frame False {
          }
          frame True {
            n244 = while {
              tunnel: [w190] -> w169
              tunnel: [w189] -> w176
              tunnel: w175 -> [w194]
              tunnel: w174 -> [w193]
              tunnel: w173 -> [w192]
              tunnel: [w191] -> w172
              tunnel: w171 -> [w187]
              tunnel: [w178] -> w170
              tunnel: [w177] -> w168
              stop <- TRUE stop-if-true
              # "READ CONTROLS SECTION"
              # "CRC READ BUTTONS"
              n245 = Multiply(x=i16 1000, y="Sample Rate (s)") -> (x*y=w185:i16)
              n246 = Subtract(x=w185, y=i16 0) -> (x-y=w183:i16)
              n247 = In Range and Coerce(upper limit=inf, x=w183, lower limit=i16 0) -> (coerced(x)=w182:dbl)  [unwired: 1 out]
              n248 = event shown="[14] \"Temperature 2 Display\": Value Change" {
                selector: _ -> [_ _ _ _ _ _ _ _ _ _ _ _ _ _ _ _ _ _ _ _ _ _ _ _ _]
                dyn-events: _ -> [_ _ _ _ _ _ _ _ _ _ _ _ _ _ _ _ _ _ _ _ _ _ _ _ _]
                timeout: w182 -> [_ _ _ _ _ _ _ _ _ _ _ _ _ _ _ _ _ _ _ _ _ _ _ _ _]
                tunnel: [w209 w222 w243 w261 w278 w300 w331 w376 w418 w455 w494 w537 w555 w570 w634 w693 w736 w783 w829 w846 w870 _ w896 w929 w957] -> w189
                tunnel: [w208 w223 w242 w260 w279 w299 w339 w377 w417 w450 w497 w534 w552 w569 w633 w691 w740 w786 w828 w845 w872 _ w897 w927 w956] -> w190
                tunnel: w194 -> [w207 _ w240 w258 w277 w305 w344 w383 w423 w463 w503 w536 w554 w572 w637 w690 w741 w787 w827 w848 w871 _ w895 w931 w956]
                tunnel: w193 -> [w206 w225 w239 w257 w276 w304 w343 w384 w424 w462 w502 w535 w553 w571 w635 w694 w739 w782 w830 w849 w873 _ w900 w926 w957]
                tunnel: w192 -> [w205 w226 w238 w256 w275 w303 w342 w382 w422 w461 w501 w533 w551 w573 w638 w695 w738 w785 w826 w850 w869 _ w901 w933 _]
                tunnel: [_ _ _ _ _ _ _ _ _ _ _ _ _ _ w632 _ _ _ _ _ _ _ _ _ _] -> w191
                tunnel: [w204 w221 w237 w255 w273 w291 w328 w369 w409 w453 w490 w532 w549 w567 w629 w688 w733 w779 w825 w844 w863 _ w889 w924 _] -> w177
                event "Output Polarity": Value Change {
                  n249 = event-data() -> ("NewVal"=w210:enum32{"Cool", "Heat "})  [unwired: 1 in, 5 out]
                  n250 = case shown="No Error" w206 {
                    selector: w206 -> [w215 w220]
                    tunnel: w210 -> [w217 _]
                    tunnel: [w216 w220] -> w209
                    tunnel: [w214 w219] -> w208
                    tunnel: w207 -> [_ w219]
                    tunnel: w205 -> [w213 _]
                    tunnel: [w211 FALSE ("End")] -> w204
                    frame No Error {
                      n251 = call "SEND COMMAND TC-48-20.vi"("Communications Port"=w213, "Format String"="21%04x", "error in"=w215, "Data"=w217) -> ("CRC ERROR"=w214:bool, "End"=w211:bool, "error out"=w216:errorcluster)  [unwired: 1 in]
                    }
                    frame Error {
                    }
                  }
                }
                event "Alarm Latch": Value Change {
                  n252 = event-data() -> ("NewVal"=w224:T1)  [unwired: 1 in, 5 out]
                  n253 = case shown="No Error" w225 {
                    selector: w225 -> [w232 w236]
                    tunnel: [w233 FALSE] -> w223
                    tunnel: [w231 w236] -> w222
                    tunnel: w226 -> [w230 _]
                    tunnel: w224 -> [w229 _]
                    tunnel: [w227 FALSE ("End")] -> w221
                    frame No Error {
                      n254 = call "SEND COMMAND TC-48-20.vi"("Communications Port"=w230, "Format String"="2b%04x", "error in"=w232, "Data"=w229) -> ("CRC ERROR"=w233:bool, "End"=w227:bool, "error out"=w231:errorcluster)  [unwired: 1 in]
                    }
                    frame Error {
                    }
                  }
                }
                event "Shutdown Output w/ Alarm 2": Value Change {
                  n255 = event-data() -> ("NewVal"=w241:bool)  [unwired: 1 in, 5 out]
                  n256 = case shown="No Error" w239 {
                    selector: w239 -> [w249 w254]
                    tunnel: [w251 w253] -> w242
                    tunnel: [w250 w254] -> w243
                    tunnel: w241 -> [w248 _]
                    tunnel: w240 -> [_ w253]
                    tunnel: w238 -> [w247 _]
                    tunnel: [w244 FALSE ("End")] -> w237
                    frame No Error {
                      n257 = Boolean To (0,1)(Boolean=w248) -> (0, 1=w245:i16)
                      n258 = call "SEND COMMAND TC-48-20.vi"("Communications Port"=w247, "Format String"="2a%04x", "error in"=w249, "Data"=w245) -> ("CRC ERROR"=w251:bool, "End"=w244:bool, "error out"=w250:errorcluster)  [unwired: 1 in]
                    }
                    frame Error {
                    }
                  }
                }
                event "Shutdown Output w/ Alarm 1": Value Change {
                  n259 = event-data() -> ("NewVal"=w259:bool)  [unwired: 1 in, 5 out]
                  n260 = case shown="No Error" w257 {
                    selector: w257 -> [w267 w272]
                    tunnel: [w269 w271] -> w260
                    tunnel: [w268 w272] -> w261
                    tunnel: w259 -> [w266 _]
                    tunnel: w258 -> [_ w271]
                    tunnel: w256 -> [w265 _]
                    tunnel: [w262 FALSE ("End")] -> w255
                    frame No Error {
                      n261 = Boolean To (0,1)(Boolean=w266) -> (0, 1=w263:i16)
                      n262 = call "SEND COMMAND TC-48-20.vi"("Communications Port"=w265, "Format String"="27%04x", "error in"=w267, "Data"=w263) -> ("CRC ERROR"=w269:bool, "End"=w262:bool, "error out"=w268:errorcluster)  [unwired: 1 in]
                    }
                    frame Error {
                    }
                  }
                }
                event "Clear Alarm Latch": Value Change {
                  n263 = event-data() -> ("OldVal"=w274:bool)  [unwired: 1 in, 5 out]
                  n264 = case shown="No Error" w276 {
                    selector: w276 -> [w286 w290]
                    tunnel: [w287 w290] -> w278
                    tunnel: [w285 w289] -> w279
                    tunnel: w277 -> [_ w289]
                    tunnel: w275 -> [w284 _]
                    tunnel: w274 -> [w282 _]
                    tunnel: [w280 FALSE ("End")] -> w273
                    frame No Error {
                      n265 = Boolean To (0,1)(Boolean=w282) -> (0, 1=w281:i16)
                      n266 = call "SEND COMMAND TC-48-20.vi"("Communications Port"=w284, "Format String"="33%04x", "error in"=w286, "Data"=w281) -> ("CRC ERROR"=w285:bool, "End"=w280:bool, "error out"=w287:errorcluster)  [unwired: 1 in]
                    }
                    frame Error {
                    }
                  }
                }
                event "Alarm 1 High": Value Change {
                  n267 = event-data() -> ("OldVal"=w297:dbl, "NewVal"=w293:dbl)  [unwired: 1 in, 4 out]
                  n268 = Greater Or Equal?(x=w293, y=200.0) -> (x >= y?=w295:bool)
                  n269 = case shown="True" w295 {
                    tunnel: [w306 200.0] -> w292
                    tunnel: w293 -> [w306 _]
                    frame False {
                    }
                    frame True {
                    }
                  }
                  n270 = case shown="No Error" w304 {
                    selector: w304 -> [w321 w327]
                    tunnel: w292 -> [w317 _]
                    tunnel: [w322 w327] -> w302
                    tunnel: [w320 w326] -> w298
                    tunnel: w305 -> [_ w326]
                    tunnel: w303 -> [w318 w324]
                    tunnel: [w317 inf] -> _
                    tunnel: [w318 w324] -> w301
                    tunnel: [w316 FALSE ("End")] -> w291
                    frame No Error {
                      n271 = call "SEND COMMAND TC-48-20.vi"("Communications Port"=w318, "Format String"="26%04x", "error in"=w321, "Data"=w317) -> ("CRC ERROR"=w320:bool, "End"=w316:bool, "error out"=w322:errorcluster)  [unwired: 1 in]
                    }
                    frame Error {
                    }
                  }
                  n272 = case shown="No Error" w302 {
                    selector: w302 -> [w311 w315]
                    tunnel: w301 -> [w312 _]
                    tunnel: [w310 w315] -> w300
                    tunnel: [w309 w314] -> w299
                    tunnel: w298 -> [_ w314]
                    tunnel: [w308 w313] -> w296
                    tunnel: w297 -> [_ w313]
                    frame No Error {
                      n273 = call "QUERY HIGH ALARM SET POINT M9613.vi"("Communications Port"=w312, "error in"=w311) -> ("CRC ERROR"=w309:bool, "HIGH ALARM SETPOINT INPUT 1"=w308:dbl, "error out"=w310:errorcluster)
                    }
                    frame Error {
                    }
                  }
                  n274 = property on="Alarm 1 High" class="DigNum (strict)"("Value"=w296) -> ()  [unwired: 2 in, 2 out]
                }
                event "Alarm 2 High": Value Change {
                  n275 = event-data() -> ("OldVal"=w337:dbl, "NewVal"=w332:dbl)  [unwired: 1 in, 4 out]
                  n276 = Greater Or Equal?(x=w332, y=200.0) -> (x >= y?=w335:bool)
                  n277 = case shown="True" w335 {
                    tunnel: [w345 200.0] -> w333
                    tunnel: w332 -> [w345 _]
                    frame False {
                    }
                    frame True {
                    }
                  }
                  n278 = case shown="No Error" w343 {
                    selector: w343 -> [w362 w367]
                    tunnel: w333 -> [w358 _]
                    tunnel: [w363 w367] -> w341
                    tunnel: [w361 w366] -> w340
                    tunnel: w344 -> [_ w366]
                    tunnel: w342 -> [w359 w365]
                    tunnel: [w359 w365] -> w336
                    tunnel: [w357 FALSE ("End")] -> w330
                    frame No Error {
                      n279 = call "SEND COMMAND TC-48-20.vi"("Communications Port"=w359, "Format String"="29%04x", "error in"=w362, "Data"=w358) -> ("CRC ERROR"=w361:bool, "End"=w357:bool, "error out"=w363:errorcluster)  [unwired: 1 in]
                    }
                    frame Error {
                    }
                  }
                  n280 = case shown="No Error" w341 {
                    selector: w341 -> [w352 w356]
                    tunnel: [w351 w356] -> w331
                    tunnel: [w350 w355] -> w339
                    tunnel: [w349 w354] -> w338
                    tunnel: w340 -> [_ w355]
                    tunnel: w337 -> [_ w354]
                    tunnel: w336 -> [w348 _]
                    tunnel: [w347 FALSE ("End")] -> w329
                    frame No Error {
                      n281 = call "QUERY HIGH ALARM SET POINT INPUT 2 M9613.vi"("Communications Port"=w348, "error in"=w352) -> ("CRC ERROR"=w350:bool, "End"=w347:bool, "HIGH ALARM SETPOINT INPUT 2"=w349:dbl, "error out"=w351:errorcluster)
                    }
                    frame Error {
                    }
                  }
                  n282 = property on="Alarm 2 High" class="DigNum (strict)"("Value"=w338) -> ()  [unwired: 2 in, 2 out]
                  n283 = Or(x=w330, y=w329) -> (x .or. y?=w328:bool)
                }
                event "Alarm 1 Low": Value Change {
                  n284 = event-data() -> ("OldVal"=w379:dbl, "NewVal"=w372:dbl)  [unwired: 1 in, 4 out]
                  n285 = Less Or Equal?(x=w372, y=-21.0) -> (x <= y?=w374:bool)
                  n286 = case shown="True" w374 {
                    tunnel: [w385 -21.0] -> w371
                    tunnel: w372 -> [w385 _]
                    frame False {
                    }
                    frame True {
                    }
                  }
                  n287 = case shown="No Error" w384 {
                    selector: w384 -> [w402 w407]
                    tunnel: w371 -> [w398 _]
                    tunnel: [w403 w407] -> w381
                    tunnel: [w401 w406] -> w378
                    tunnel: w383 -> [_ w406]
                    tunnel: w382 -> [w399 w405]
                    tunnel: [w399 w405] -> w375
                    tunnel: [w397 FALSE ("End")] -> w370
                    frame No Error {
                      n288 = call "SEND COMMAND TC-48-20.vi"("Communications Port"=w399, "Format String"="25%04x", "error in"=w402, "Data"=w398) -> ("CRC ERROR"=w401:bool, "End"=w397:bool, "error out"=w403:errorcluster)  [unwired: 1 in]
                    }
                    frame Error {
                    }
                  }
                  n289 = case shown="No Error" w381 {
                    selector: w381 -> [w392 w396]
                    tunnel: [w391 w396] -> w376
                    tunnel: [w390 w394] -> w377
                    tunnel: [w389 w395] -> w380
                    tunnel: w379 -> [_ w395]
                    tunnel: w378 -> [_ w394]
                    tunnel: w375 -> [w388 _]
                    tunnel: [w387 FALSE ("End")] -> w368
                    frame No Error {
                      n290 = call "QUERY LOW ALARM SET POINT M9613.vi"("Communications Port"=w388, "error in"=w392) -> ("CRC ERROR"=w390:bool, "End"=w387:bool, "LOW ALARM SETPOINT"=w389:dbl, "error out"=w391:errorcluster)
                    }
                    frame Error {
                    }
                  }
                  n291 = property on="Alarm 2 Low" class="DigNum (strict)"("Value"=w380) -> ()  [unwired: 2 in, 2 out]
                  n292 = Or(x=w370, y=w368) -> (x .or. y?=w369:bool)
                }
                event "Alarm 2 Low": Value Change {
                  n293 = event-data() -> ("OldVal"=w419:dbl, "NewVal"=w412:dbl)  [unwired: 1 in, 4 out]
                  n294 = Less Or Equal?(x=w412, y=-21) -> (x <= y?=w414:bool)
                  n295 = case shown="False" w414 {
                    tunnel: [w425 -21] -> w411
                    tunnel: w412 -> [w425 _]
                    frame False {
                    }
                    frame True {
                    }
                  }
                  n296 = case shown="No Error" w424 {
                    selector: w424 -> [w443 w449]
                    tunnel: w411 -> [w445 _]
                    tunnel: [w444 w449] -> w421
                    tunnel: [w442 w448] -> w420
                    tunnel: w423 -> [_ w448]
                    tunnel: w422 -> [w438 w447]
                    tunnel: [w438 w447] -> w416
                    tunnel: [w437 FALSE ("End")] -> w410
                    frame No Error {
                      n297 = Multiply(x=1, y=w445) -> (x*y=w440:dbl)
                      n298 = call "SEND COMMAND TC-48-20.vi"("Communications Port"=w438, "Format String"="28%04x", "error in"=w443, "Data"=w440) -> ("CRC ERROR"=w442:bool, "End"=w437:bool, "error out"=w444:errorcluster)  [unwired: 1 in]
                    }
                    frame Error {
                    }
                  }
                  n299 = case shown="No Error" w421 {
                    selector: w421 -> [w432 w436]
                    tunnel: [w431 w436] -> w418
                    tunnel: [w430 w435] -> w417
                    tunnel: [w429 w434] -> w415
                    tunnel: w420 -> [_ w435]
                    tunnel: w419 -> [_ w434]
                    tunnel: w416 -> [w428 _]
                    tunnel: [w427 FALSE ("End")] -> w408
                    frame No Error {
                      n300 = call "QUERY LOW ALARM SET POINT INPUT 2 M9613.vi"("Communications Port"=w428, "error in"=w432) -> ("CRC ERROR"=w430:bool, "End"=w427:bool, "LOW ALARM SETPOINT INPUT 2"=w429:dbl, "error out"=w431:errorcluster)
                    }
                    frame Error {
                    }
                  }
                  n301 = property on="Alarm 2 Low" class="DigNum (strict)"("Value"=w415) -> ()  [unwired: 2 in, 2 out]
                  n302 = Or(x=w410, y=w408) -> (x .or. y?=w409:bool)
                }
                event "Alarm 1 Deadband": Value Change {
                  n303 = event-data() -> ("NewVal"=w464:dbl)  [unwired: 1 in, 5 out]
                  n304 = Multiply(x=w464, y=10) -> (x*y=w456:dbl)
                  n305 = case shown="No Error" w462 {
                    selector: w462 -> [w483 w489]
                    tunnel: w456 -> [w485 _]
                    tunnel: [w484 w489] -> w459
                    tunnel: [w482 w488] -> w458
                    tunnel: w463 -> [_ w488]
                    tunnel: w461 -> [w480 w487]
                    tunnel: [w480 w487] -> w457
                    tunnel: [w479 FALSE ("End")] -> w454
                    frame No Error {
                      n306 = call "SEND COMMAND TC-48-20.vi"("Communications Port"=w480, "Format String"="2d%04x", "error in"=w483, "Data"=w485) -> ("CRC ERROR"=w482:bool, "End"=w479:bool, "error out"=w484:errorcluster)  [unwired: 1 in]
                    }
                    frame Error {
                    }
                  }
                  n307 = case shown="No Error" w459 {
                    selector: w459 -> [w476 w478]
                    tunnel: w457 -> [w475 _]
                    tunnel: [w473 w478] -> w455
                    tunnel: w456 -> [w467 _]
                    tunnel: [w472 w477] -> w452
                    tunnel: [w471 w477] -> w451
                    frame No Error {
                      n308 = call "QUERY ALARM 1 DEADBAND M9613.vi"("Communications Port"=w475, "error in"=w476) -> ("CRC ERROR"=w471:bool, "End"=w472:bool, "ALARM 1 DEADBAND"=w466:dbl, "error out"=w474:errorcluster)
                      n309 = Subtract(x=w466, y=w467) -> (x-y=w470:dbl)
                      n310 = Absolute Value(x=w470) -> (abs(x)=w469:dbl)
                      n311 = Greater?(x=w469, y=0.01) -> (0:w465:bool)
                      n312 = Bundle By Name(cluster=w474, "status"=w465) -> (w473:errorcluster)
                    }
                    frame Error {
                      w477 = FALSE ("End")
                    }
                  }
                  n313 = Or(x=w454, y=w452) -> (x .or. y?=w453:bool)
                  n314 = Or(x=w458, y=w451) -> (x .or. y?=w450:bool)
                }
                event "Alarm 2 Deadband": Value Change {
                  n315 = event-data() -> ("NewVal"=w504:dbl)  [unwired: 1 in, 5 out]
                  n316 = Multiply(x=w504, y=10) -> (x*y=w500:dbl)
                  n317 = case shown="Error" w502 {
                    selector: w502 -> [w525 w531]
                    tunnel: w500 -> [w521 w528]
                    tunnel: [w526 w531] -> w498
                    tunnel: [w524 w530] -> w496
                    tunnel: w503 -> [_ w530]
                    tunnel: w501 -> [w522 w529]
                    tunnel: [w522 w529] -> w495
                    tunnel: [w521 w528] -> w493
                    tunnel: [w520 FALSE ("End")] -> w492
                    frame No Error {
                      n318 = call "SEND COMMAND TC-48-20.vi"("Communications Port"=w522, "Format String"="2e%04x", "error in"=w525, "Data"=w521) -> ("CRC ERROR"=w524:bool, "End"=w520:bool, "error out"=w526:errorcluster)  [unwired: 1 in]
                    }
                    frame Error {
                    }
                  }
                  n319 = case shown="No Error" w498 {
                    selector: w498 -> [w516 w518]
                    tunnel: [w515 w519] -> w497
                    tunnel: w496 -> [_ w519]
                    tunnel: w495 -> [w514 _]
                    tunnel: [w512 w518] -> w494
                    tunnel: w493 -> [w507 _]
                    tunnel: [w511 FALSE ("END")] -> w491
                    frame No Error {
                      n320 = call "QUERY ALARM 2 DEADBAND M9613.vi"("error in"=w516, "Communications Port"=w514) -> ("error out"=w513:errorcluster, "ALARM 2 DEADBAND"=w506:dbl, "END"=w511:bool, "CRC ERROR"=w515:bool)  [unwired: 1 in]
                      n321 = Subtract(x=w506, y=w507) -> (x-y=w510:dbl)
                      n322 = Absolute Value(x=w510) -> (abs(x)=w509:dbl)
                      n323 = Greater?(x=w509, y=0.01) -> (0:w505:bool)
                      n324 = Bundle By Name(cluster=w513, "status"=w505) -> (w512:errorcluster)
                    }
                    frame Error {
                    }
                  }
                  n325 = Or(x=w492, y=w491) -> (x .or. y?=w490:bool)
                }
                event "Sensor Type": Value Change {
                  n326 = event-data() -> ("NewVal"=w538:enum32{"15K", "10K"})  [unwired: 1 in, 5 out]
                  n327 = case shown="No Error" w535 {
                    selector: w535 -> [w542 w548]
                    tunnel: [w544 w548] -> w537
                    tunnel: [w543 w547] -> w534
                    tunnel: w538 -> [w541 _]
                    tunnel: w536 -> [_ w547]
                    tunnel: w533 -> [w540 _]
                    tunnel: [w539 FALSE ("End")] -> w532
                    frame No Error {
                      n328 = call "SEND COMMAND TC-48-20.vi"("Communications Port"=w540, "Format String"="20%04x", "error in"=w542, "Data"=w541) -> ("CRC ERROR"=w543:bool, "End"=w539:bool, "error out"=w544:errorcluster)  [unwired: 1 in]
                    }
                    frame Error {
                    }
                  }
                }
                event "Run Peltier": Value Change {
                  n329 = event-data() -> ("NewVal"=w556:bool)  [unwired: 1 in, 5 out]
                  n330 = Boolean To (0,1)(Boolean=w556) -> (0, 1=w550:i16)
                  n331 = case shown="Error" w553 {
                    selector: w553 -> [w560 w566]
                    tunnel: [w562 w566] -> w555
                    tunnel: [w561 w565] -> w552
                    tunnel: w550 -> [w559 _]
                    tunnel: w554 -> [_ w565]
                    tunnel: w551 -> [w558 _]
                    tunnel: [w557 FALSE ("End")] -> w549
                    frame No Error {
                      n332 = call "SEND COMMAND TC-48-20.vi"("Communications Port"=w558, "Format String"="30%04x", "error in"=w560, "Data"=w559) -> ("CRC ERROR"=w561:bool, "End"=w557:bool, "error out"=w562:errorcluster)  [unwired: 1 in]
                    }
                    frame Error {
                    }
                  }
                }
                event "Set Temperature": Value Change {
                  n333 = event-data() -> ("NewVal"=w568:dbl)  [unwired: 1 in, 5 out]
                  n334 = case shown="No Error" w571 {
                    selector: w571 -> [w593 w627]
                    tunnel: w572 -> [w584 w626]
                    tunnel: w573 -> [w590 _]
                    tunnel: w568 -> [w582 _]
                    tunnel: [w591 w627] -> w570
                    tunnel: [w585 w626] -> w569
                    tunnel: [w576 FALSE ("End")] -> w567
                    frame No Error {
                      n335 = property on="Set Limit High" class="DigNum (strict)"() -> ("Value"=w578:dbl)  [unwired: 2 in, 2 out]
                      n336 = Greater Or Equal?(x=w582, y=w578) -> (x >= y?=w583:bool)
                      n337 = case shown="True" w583 {
                        tunnel: [w596 w597] -> w580
                        tunnel: w582 -> [w596 _]
                        tunnel: w578 -> [_ w597]
                        frame False {
                        }
                        frame True {
                        }
                      }
                      n338 = property on="Set Limit Low" class="DigNum (strict)"() -> ("Value"=w577:dbl)  [unwired: 2 in, 2 out]
                      n339 = Less Or Equal?(x=w580, y=w577) -> (x <= y?=w581:bool)
                      n340 = case shown="False" w581 {
                        tunnel: [w594 w595] -> w579
                        tunnel: w580 -> [w594 _]
                        tunnel: w577 -> [_ w595]
                        frame False {
                        }
                        frame True {
                        }
                      }
                      n341 = Multiply(x=10, y=w579) -> (x*y=w589:dbl)
                      n342 = case shown="No Error" w593 {
                        selector: w593 -> [w620 w624]
                        tunnel: [w621 w624] -> w592
                        tunnel: [w619 w623] -> w587
                        tunnel: w584 -> [_ w623]
                        tunnel: w590 -> [w618 _]
                        tunnel: w589 -> [w616 _]
                        tunnel: [w615 FALSE ("End")] -> w574
                        frame No Error {
                          n343 = call "SEND COMMAND TC-48-20.vi"("Communications Port"=w618, "Format String"="1c%04x", "error in"=w620, "Data"=w616) -> ("CRC ERROR"=w619:bool, "End"=w615:bool, "error out"=w621:errorcluster)  [unwired: 1 in]
                        }
                        frame Error {
                        }
                      }
                      n344 = case shown="No Error" w592 {
                        selector: w592 -> [w605 w614]
                        tunnel: [w608 w612] -> w591
                        tunnel: [w609 TRUE] -> w586
                        tunnel: w590 -> [w606 _]
                        tunnel: w579 -> [w600 _]
                        tunnel: [w598 FALSE ("End")] -> w575
                        frame No Error {
                          n345 = call "QUERY SETPOINT M9613.vi"("Communications Port"=w606, "error in"=w605) -> ("CRC ERROR"=w609:bool, "End"=w598:bool, "SET POINT"=w599:dbl, "error out"=w607:errorcluster)
                          n346 = Subtract(x=w599, y=w600) -> (x-y=w604:dbl)
                          n347 = Absolute Value(x=w604) -> (abs(x)=w603:dbl)
                          n348 = Greater?(x=w603, y=0.01) -> (0:w601:bool)
                          n349 = Bundle By Name(cluster=w607, "status"=w601) -> (w608:errorcluster)
                        }
                        frame Error {
                          n350 = call <vilib>:"Simple Error Handler.vi"("error source (\" \")"="SET TEMPERATURE ERROR", "error in (no error)"=w614) -> ("error out"=w612:errorcluster)  [unwired: 3 in, 4 out]
                        }
                      }
                      n351 = Or(x=w574, y=w575) -> (x .or. y?=w576:bool)
                      n352 = Compound Arithmetic op=OR(w587, w586) -> (w585:bool)
                    }
                    frame Error {
                    }
                  }
                }
                event "Temperature 2 Display": Value Change {
                  n353 = event-data() -> ("OldVal"=w631:T3, "NewVal"=w636:T3)  [unwired: 1 in, 4 out]
                  n354 = case shown="No Error" w635 {
                    selector: w635 -> [w652 w686]
                    tunnel: w637 -> [w653 w685]
                    tunnel: w638 -> [w649 _]
                    tunnel: w636 -> [w646 _]
                    tunnel: [w650 w686] -> w634
                    tunnel: [w643 w685] -> w633
                    tunnel: [w642 0] -> w632
                    tunnel: w631 -> [w641 _]
                    tunnel: [w639 FALSE ("End")] -> w628
                    tunnel: [w640 FALSE ("End")] -> w630
                    frame No Error {
                      n355 = Multiply(x=1.0 ("y"), y=w646) -> (x*y=w648:dbl)
                      n356 = case shown="Error" w652 {
                        selector: w652 -> [w677 w681]
                        tunnel: [w678 w681] -> w651
                        tunnel: [w676 w680] -> w645
                        tunnel: w653 -> [_ w680]
                        tunnel: w649 -> [w675 _]
                        tunnel: w648 -> [w673 _]
                        tunnel: [w672 FALSE ("End")] -> w639
                        frame No Error {
                          n357 = call "SEND COMMAND TC-48-20.vi"("Communications Port"=w675, "Format String"="2c%04x", "error in"=w677, "Data"=w673) -> ("CRC ERROR"=w676:bool, "End"=w672:bool, "error out"=w678:errorcluster)  [unwired: 1 in]
                        }
                        frame Error {
                        }
                      }
                      n358 = case shown="No Error" w651 {
                        selector: w651 -> [w661 w671]
                        tunnel: [w664 w669] -> w650
                        tunnel: [w665 TRUE] -> w644
                        tunnel: w649 -> [w662 _]
                        tunnel: w646 -> [w655 _]
                        tunnel: [w656 w667] -> w642
                        tunnel: w641 -> [_ w667]
                        tunnel: [w660 FALSE ("End")] -> w640
                        frame No Error {
                          n359 = call "QUERY TEMP 2 DISPLAY M9613.vi"("Communications Port"=w662, "error in"=w661) -> ("CRC ERROR"=w665:bool, "End"=w660:bool, "TEMPERATURE 2 DISPLAY"=w656:dbl, "error out"=w663:errorcluster)
                          n360 = Subtract(x=w655, y=w656) -> (x-y=w659:dbl)
                          n361 = Absolute Value(x=w659) -> (abs(x)=w658:dbl)
                          n362 = Greater?(x=w658, y=0.01) -> (0:w654:bool)
                          n363 = Bundle By Name(cluster=w663, "status"=w654) -> (w664:errorcluster)
                        }
                        frame Error {
                          n364 = call <vilib>:"Simple Error Handler.vi"("error source (\" \")"="SET TEMPERATURE ERROR", "error in (no error)"=w671) -> ("error out"=w669:errorcluster)  [unwired: 3 in, 4 out]
                        }
                      }
                      n365 = Or(x=w645, y=w644) -> (x .or. y?=w643:bool)
                    }
                    frame Error {
                    }
                  }
                  n366 = Or(x=w628, y=w630) -> (x .or. y?=w629:bool)
                }
                event "Proportional Bandwidth": Value Change {
                  n367 = event-data() -> ("NewVal"=w692:dbl)  [unwired: 1 in, 5 out]
                  n368 = case shown="No Error" w694 {
                    selector: w694 -> [w701 w732]
                    tunnel: [w703 w728] -> w691
                    tunnel: [w704 w731] -> w693
                    tunnel: w695 -> [w698 _]
                    tunnel: w692 -> [w699 _]
                    tunnel: w690 -> [_ w728]
                    tunnel: [w697 w727] -> w689
                    tunnel: [w696 w727] -> w687
                    frame No Error {
                      n369 = case shown="No Error" w701 {
                        selector: w701 -> [w721 w726]
                        tunnel: [w723 w726] -> w700
                        tunnel: [w720 TRUE] -> w705
                        tunnel: w698 -> [w719 _]
                        tunnel: w699 -> [w717 _]
                        tunnel: [w715 FALSE ("End")] -> w697
                        frame No Error {
                          n370 = Multiply(x=w717, y=10) -> (x*y=w716:dbl)
                          n371 = call "SEND COMMAND TC-48-20.vi"("Communications Port"=w719, "Format String"="1d%04x", "error in"=w721, "Data"=w716) -> ("CRC ERROR"=w720:bool, "End"=w715:bool, "error out"=w723:errorcluster)  [unwired: 1 in]
                        }
                        frame Error {
                        }
                      }
                      n372 = case shown="No Error" w700 {
                        selector: w700 -> [w709 w714]
                        tunnel: [w708 w714] -> w704
                        tunnel: [w711 TRUE] -> w702
                        tunnel: w698 -> [w710 _]
                        tunnel: [w706 FALSE ("End")] -> w696
                        frame No Error {
                          n373 = call "QUERY PROPORTIONAL BW M9613.vi"("Communications Port"=w710, "error in"=w709) -> ("CRC ERROR"=w711:bool, "End"=w706:bool, "PROPOTIONAL BW"=w707:dbl, "error out"=w708:errorcluster)
                          n374 = property on="Proportional Bandwidth" class="DigNum (strict)"("Value"=w707) -> ()  [unwired: 2 in, 2 out]
                        }
                        frame Error {
                        }
                      }
                      n375 = Or(x=w705, y=w702) -> (x .or. y?=w703:bool)
                    }
                    frame Error {
                      w727 = FALSE ("End")
                      w729 = T7 2 items=["no dialog", "OK message", "continue or stop message", "OK message + warnings", "continue/stop + warnings"] ("type of dialog (OK msg:1)")
                      n376 = call <vilib>:"Simple Error Handler.vi"("error source (\" \")"="PROPORTIONAL SEND ERROR", "type of dialog (OK msg:1)"=w729, "error in (no error)"=w732) -> ("error out"=w731:errorcluster)  [unwired: 2 in, 4 out]
                    }
                  }
                  n377 = Or(x=w689, y=w687) -> (x .or. y?=w688:bool)
                }
                event "Integral Gain": Value Change {
                  n378 = event-data() -> ("NewVal"=w737:dbl)  [unwired: 1 in, 5 out]
                  n379 = case shown="No Error" w739 {
                    selector: w739 -> [w747 w778]
                    tunnel: [w749 w774] -> w740
                    tunnel: [w750 w777] -> w736
                    tunnel: w738 -> [w744 _]
                    tunnel: w737 -> [w745 _]
                    tunnel: w741 -> [_ w774]
                    tunnel: [w743 w773] -> w734
                    tunnel: [w742 w773] -> w735
                    frame No Error {
                      n380 = case shown="No Error" w747 {
                        selector: w747 -> [w767 w772]
                        tunnel: [w769 w772] -> w746
                        tunnel: [w766 TRUE] -> w751
                        tunnel: w744 -> [w765 _]
                        tunnel: w745 -> [w763 _]
                        tunnel: [w761 FALSE ("End")] -> w743
                        frame No Error {
                          n381 = Multiply(x=w763, y=100) -> (x*y=w764:dbl)
                          n382 = call "SEND COMMAND TC-48-20.vi"("Communications Port"=w765, "Format String"="1e%04x", "error in"=w767, "Data"=w764) -> ("CRC ERROR"=w766:bool, "End"=w761:bool, "error out"=w769:errorcluster)  [unwired: 1 in]
                        }
                        frame Error {
                        }
                      }
                      n383 = case shown="No Error" w746 {
                        selector: w746 -> [w755 w760]
                        tunnel: [w754 w760] -> w750
                        tunnel: [w757 TRUE] -> w748
                        tunnel: w744 -> [w756 _]
                        tunnel: [w752 FALSE ("End")] -> w742
                        frame No Error {
                          n384 = call "QUERY INTEGRAL GAIN M9613.vi"("Communications Port"=w756, "error in"=w755) -> ("CRC ERROR"=w757:bool, "End"=w752:bool, "INTEGRAL GAIN"=w753:dbl, "error out"=w754:errorcluster)
                          n385 = property on="Integral Gain" class="DigNum (strict)"("Value"=w753) -> ()  [unwired: 2 in, 2 out]
                        }
                        frame Error {
                        }
                      }
                      n386 = Or(x=w751, y=w748) -> (x .or. y?=w749:bool)
                    }
                    frame Error {
                      w773 = FALSE ("End")
                      w775 = T7 2 items=["no dialog", "OK message", "continue or stop message", "OK message + warnings", "continue/stop + warnings"] ("type of dialog (OK msg:1)")
                      n387 = call <vilib>:"Simple Error Handler.vi"("error source (\" \")"="INTEGRAL ERROR", "type of dialog (OK msg:1)"=w775, "error in (no error)"=w778) -> ("error out"=w777:errorcluster)  [unwired: 2 in, 4 out]
                    }
                  }
                  n388 = Or(x=w734, y=w735) -> (x .or. y?=w733:bool)
                }
                event "Derivative Gain": Value Change {
                  n389 = event-data() -> ("NewVal"=w784:dbl)  [unwired: 1 in, 5 out]
                  n390 = case shown="No Error" w782 {
                    selector: w782 -> [w793 w824]
                    tunnel: [w795 w820] -> w786
                    tunnel: [w796 w823] -> w783
                    tunnel: w785 -> [w790 _]
                    tunnel: w784 -> [w791 _]
                    tunnel: w787 -> [_ w820]
                    tunnel: [w789 w819] -> w781
                    tunnel: [w788 w819] -> w780
                    frame No Error {
                      n391 = case shown="No Error" w793 {
                        selector: w793 -> [w813 w818]
                        tunnel: [w815 w818] -> w792
                        tunnel: [w812 TRUE] -> w797
                        tunnel: w790 -> [w811 _]
                        tunnel: w791 -> [w810 _]
                        tunnel: [w807 FALSE ("End")] -> w789
                        frame No Error {
                          n392 = Multiply(x=w810, y=100) -> (x*y=w808:dbl)
                          n393 = call "SEND COMMAND TC-48-20.vi"("Communications Port"=w811, "Format String"="1f%04x", "error in"=w813, "Data"=w808) -> ("CRC ERROR"=w812:bool, "End"=w807:bool, "error out"=w815:errorcluster)  [unwired: 1 in]
                        }
                        frame Error {
                        }
                      }
                      n394 = case shown="No Error" w792 {
                        selector: w792 -> [w800 w806]
                        tunnel: [w801 w806] -> w796
                        tunnel: [w803 TRUE] -> w794
                        tunnel: w790 -> [w802 _]
                        tunnel: [w798 FALSE ("End")] -> w788
                        frame No Error {
                          n395 = call "QUERY DERIVATIVE GAIN M9613.vi"("Communications Port"=w802, "error in"=w800) -> ("CRC ERROR"=w803:bool, "End"=w798:bool, "DERIVATIVE GAIN"=w799:dbl, "error out"=w801:errorcluster)
                          n396 = property on="Derivative Gain" class="DigNum (strict)"("Value"=w799) -> ()  [unwired: 2 in, 2 out]
                        }
                        frame Error {
                        }
                      }
                      n397 = Or(x=w797, y=w794) -> (x .or. y?=w795:bool)
                    }
                    frame Error {
                      w819 = FALSE ("End")
                      w821 = T7 2 items=["no dialog", "OK message", "continue or stop message", "OK message + warnings", "continue/stop + warnings"] ("type of dialog (OK msg:1)")
                      n398 = call <vilib>:"Simple Error Handler.vi"("error source (\" \")"="DERATIVE ERROR", "type of dialog (OK msg:1)"=w821, "error in (no error)"=w824) -> ("error out"=w823:errorcluster)  [unwired: 2 in, 4 out]
                    }
                  }
                  n399 = Or(x=w781, y=w780) -> (x .or. y?=w779:bool)
                }
                event "Set Limit High": Value Change {
                  n400 = event-data() -> ("NewVal"=w831:dbl)  [unwired: 1 in, 5 out]
                  n401 = Multiply(x=1, y=w831) -> (x*y=w833:dbl)
                  n402 = case shown="No Error" w830 {
                    selector: w830 -> [w839 w843]
                    tunnel: [w840 w843] -> w829
                    tunnel: [w838 w842] -> w828
                    tunnel: w833 -> [w836 _]
                    tunnel: w827 -> [_ w842]
                    tunnel: w826 -> [w835 _]
                    tunnel: [w834 FALSE ("End")] -> w825
                    frame No Error {
                      n403 = call "SEND COMMAND TC-48-20.vi"("Communications Port"=w835, "Format String"="23%04x", "error in"=w839, "Data"=w836) -> ("CRC ERROR"=w838:bool, "End"=w834:bool, "error out"=w840:errorcluster)  [unwired: 1 in]
                    }
                    frame Error {
                    }
                  }
                }
                event "Set Limit Low": Value Change {
                  n404 = event-data() -> ("NewVal"=w847:dbl)  [unwired: 1 in, 5 out]
                  n405 = Multiply(x=1, y=w847) -> (x*y=w852:dbl)
                  n406 = case shown="No Error" w849 {
                    selector: w849 -> [w858 w862]
                    tunnel: [w859 w862] -> w846
                    tunnel: [w857 w861] -> w845
                    tunnel: w848 -> [_ w861]
                    tunnel: w850 -> [w856 _]
                    tunnel: w852 -> [w854 _]
                    tunnel: [w853 FALSE ("End")] -> w844
                    frame No Error {
                      n407 = call "SEND COMMAND TC-48-20.vi"("Communications Port"=w856, "Format String"="22%04x", "error in"=w858, "Data"=w854) -> ("CRC ERROR"=w857:bool, "End"=w853:bool, "error out"=w859:errorcluster)  [unwired: 1 in]
                    }
                    frame Error {
                    }
                  }
                }
                event "Analog Output Multiplier": Value Change {
                  w867 = 100
                  n408 = event-data() -> ("NewVal"=w865:dbl)  [unwired: 1 in, 5 out]
                  n409 = Absolute Value(x=w865) -> (abs(x)=w864:dbl)
                  n410 = Greater Or Equal?(x=w864, y=w867) -> (x >= y?=w868:bool)
                  n411 = case shown="True" w868 {
                    tunnel: w867 -> [_ w875]
                    tunnel: [w874 w875] -> w866
                    tunnel: w864 -> [w874 _]
                    frame False {
                    }
                    frame True {
                    }
                  }
                  n412 = case shown="No Error" w873 {
                    selector: w873 -> [w883 w887]
                    tunnel: [w884 w887] -> w870
                    tunnel: [w882 w886] -> w872
                    tunnel: w866 -> [w879 _]
                    tunnel: w871 -> [_ w886]
                    tunnel: w869 -> [w880 _]
                    tunnel: [w876 FALSE ("End")] -> w863
                    frame No Error {
                      n413 = Multiply(x=w879, y=100) -> (x*y=w877:dbl)
                      n414 = call "SEND COMMAND TC-48-20.vi"("Communications Port"=w880, "Format String"="2f%04x", "error in"=w883, "Data"=w877) -> ("CRC ERROR"=w882:bool, "End"=w876:bool, "error out"=w884:errorcluster)  [unwired: 1 in]
                    }
                    frame Error {
                    }
                  }
                }
                event "About": Value Change {
                  n415 = event-data() -> ()  [unwired: 1 in, 6 out]
                  n416 = One Button Dialog(message="TE Technology, Inc.\nTC-48-20 Thermoelectric Temperature Controller\nRevision 1.0 (2/26/2015)") -> ()  [unwired: 1 in, 1 out]
                }
                event "Control Sensor Offset": Value Change {
                  n417 = event-data() -> ("NewVal"=w902:dbl)  [unwired: 1 in, 5 out]
                  n418 = Multiply(x=w902, y=10) -> (x*y=w893:dbl)
                  n419 = case shown="No Error" w900 {
                    selector: w900 -> [w917 w922]
                    tunnel: [w918 w922] -> w899
                    tunnel: [w916 w921] -> w894
                    tunnel: w893 -> [w914 _]
                    tunnel: w895 -> [_ w921]
                    tunnel: w901 -> [w913 w920]
                    tunnel: [w913 w920] -> w898
                    tunnel: [w912 FALSE ("End")] -> w891
                    frame No Error {
                      n420 = call "SEND COMMAND TC-48-20.vi"("Communications Port"=w913, "Format String"="24%04x", "error in"=w917, "Data"=w914) -> ("CRC ERROR"=w916:bool, "End"=w912:bool, "error out"=w918:errorcluster)  [unwired: 1 in]
                    }
                    frame Error {
                    }
                  }
                  n421 = case shown="No Error" w899 {
                    selector: w899 -> [w907 w911]
                    tunnel: w898 -> [w908 _]
                    tunnel: [w906 w910] -> w897
                    tunnel: [w905 w911] -> w896
                    tunnel: w894 -> [_ w910]
                    tunnel: [w903 FALSE ("End")] -> w890
                    frame No Error {
                      n422 = call "INPUT 1 SENSOR OFFSET M9613.vi"("Communications Port"=w908, "error in"=w907) -> ("CRC ERROR"=w906:bool, "End"=w903:bool, "INPUT 1 SENSOR OFFSET"=w904:dbl, "error out"=w905:errorcluster)
                      n423 = property on="Control Sensor Offset" class="DigNum (strict)"("Value"=w904) -> ()  [unwired: 2 in, 2 out]
                    }
                    frame Error {
                    }
                  }
                  n424 = Or(x=w891, y=w890) -> (x .or. y?=w889:bool)
                }
                event "EEPROM Write Enable": Value Change {
                  n425 = event-data() -> ("NewVal"=w934:bool)  [unwired: 1 in, 5 out]
                  n426 = Boolean To (0,1)(Boolean=w934) -> (0, 1=w935:i16)
                  n427 = case shown="No Error" w926 {
                    selector: w926 -> [w950 w955]
                    tunnel: [w951 w955] -> w932
                    tunnel: [w946 w954] -> w928
                    tunnel: w935 -> [w948 _]
                    tunnel: w931 -> [_ w954]
                    tunnel: w933 -> [w947 w953]
                    tunnel: [w947 w953] -> w930
                    tunnel: [w945 FALSE ("End")] -> w925
                    frame No Error {
                      n428 = call "SEND COMMAND TC-48-20.vi"("Communications Port"=w947, "Format String"="31%04x", "error in"=w950, "Data"=w948) -> ("CRC ERROR"=w946:bool, "End"=w945:bool, "error out"=w951:errorcluster)  [unwired: 1 in]
                    }
                    frame Error {
                    }
                  }
                  n429 = case shown="No Error" w932 {
                    selector: w932 -> [w940 w944]
                    tunnel: w930 -> [w941 _]
                    tunnel: [w939 w944] -> w929
                    tunnel: w928 -> [_ w943]
                    tunnel: [w937 w943] -> w927
                    tunnel: [w936 FALSE ("End")] -> w923
                    frame No Error {
                      n430 = call "QUERY EEPROM WRITE ENABLE.vi"("Communications Port"=w941, "error IO"=w940) -> ("EEPROM WRITE\nENABLED"=w938:bool, "End"=w936:bool, "CRC"=w937:bool, "error IO 2"=w939:errorcluster)
                      n431 = property on="EEPROM Write Enable" class="Bool (strict)"("Value"=w938) -> ()  [unwired: 2 in, 2 out]
                    }
                    frame Error {
                    }
                  }
                  n432 = Or(x=w925, y=w923) -> (x .or. y?=w924:bool)
                }
                event Timeout {
                  n433 = event-data() -> ()  [unwired: 1 in, 3 out]
                }
              }
              n434 = case shown="Error" w189 {
                tunnel: w187 -> [w200 w203]
                tunnel: [w200 w202] -> w188
                frame No Error {
                }
                frame Error {
                  w201 = TRUE
                  n435 = Bundle By Name(cluster=w203, "Read Model"=w201, "Read Settings"=w201) -> (w202:T4)
                }
              }
              n436 = case shown="True" w190 {
                selector: w190 -> [_ w197]
                tunnel: w188 -> [w196 w199]
                tunnel: [w196 w198] -> w178
                frame False {
                }
                frame True {
                  n437 = Bundle By Name(cluster=w199, "Read Model"=w197, "Read Settings"=w197) -> (w198:T4)
                }
              }
            }
          }
        }
      }
      frame Error {
      }
    }
    n438 = feedback-in #1(w92) -> ()
    n439 = case shown="True" w72 {
      selector: w72 -> [_ w104]
      tunnel: [w101 w102] -> _
      tunnel: [w101 w103] -> w68
      tunnel: w71 -> [w101 w102]
      frame False {
      }
      frame True {
        n440 = Bundle By Name(cluster=w102, "CRC Error"=w104) -> (w103:T4)
      }
    }
    n441 = case shown="True" w66 {
      selector: w66 -> [_ w99]
      tunnel: w68 -> [w97 w100]
      tunnel: [w97 w98] -> w67
      frame False {
      }
      frame True {
        n442 = Bundle By Name(cluster=w100, "End"=w99) -> (w98:T4)
      }
    }
    n443 = case shown="Error" w88 {
      selector: w88 -> [w137 w139]
      tunnel: w67 -> [w138 w142]
      tunnel: [w138 w141] -> w70
      tunnel: [w137 w139] -> w82
      frame No Error {
      }
      frame Error {
        n444 = Two Button Dialog(message=" Unable to communicate with controller (Error 3), check:\n• Controller is ON and correctly wired\n• Correct communications port is selected\n• Another program is not using the communications port ", 1:"EXIT" ("F button name (\"Cancel\")"), 2:"RESTART" ("T button name (\"OK\")")) -> (T button?=w140:bool)
        n445 = case shown="False" w140 {
          selector: w140 -> [w148 _]
          tunnel: w142 -> [w146 w150]
          tunnel: [w147 w152] -> w141
          frame False {
            n446 = Not(x=w148) -> (.not. x?=w149:bool)
            n447 = Bundle By Name(cluster=w146, "End"=w149) -> (w147:T4)
          }
          frame True {
            w151 = TRUE
            n448 = Bundle By Name(cluster=w150, "Read Model"=w151, "Read Settings"=w151, "Read Controls"=w151, "Sample"=w151, "Start"=w151) -> (w152:T4)
          }
        }
      }
    }
    "error out" <- w82
    n449 = Unbundle By Name(w70) -> ("CRC Error"=w69:bool)
    "CRC Error" <- w69
    n450 = case shown="True" w69 {
      selector: w69 -> [_ w1255]
      tunnel: [w1252 w1253] -> w64
      tunnel: w70 -> [w1252 w1254]
      frame False {
      }
      frame True {
        n451 = while {
          tunnel: w1255 -> [_]
          tunnel: w1254 -> [w1257]
          tunnel: [w1256] -> w1253
          stop <- TRUE stop-if-true
          n452 = Two Button Dialog(message="COMMUNICATIONS\nERROR, CONTINUE?", 1:"STOP", 2:"CONTINUE") -> (T button?=w1258:bool)
          n453 = case shown="False" w1258 {
            selector: w1258 -> [w1265 _]
            tunnel: w1257 -> [w1263 w1268]
            tunnel: [w1264 w1270] -> w1256
            frame False {
              n454 = Not(x=w1265) -> (.not. x?=w1266:bool)
              n455 = Bundle By Name(cluster=w1263, "End"=w1266) -> (w1264:T4)
            }
            frame True {
              w1269 = TRUE
              n456 = Bundle By Name(cluster=w1268, "Read Model"=w1269, "Read Settings"=w1269, "Read Controls"=w1269, "Sample"=FALSE, "Start"=w1269) -> (w1270:T4)
            }
          }
        }
      }
    }
    n457 = Unbundle By Name(w64) -> ("End"=w77:bool)
  }
